vi "MC_7_23a_JW.vi"() -> ()   [LabVIEW 2011]
uses:
  <vilib>/Utility/file.llb/Read From Spreadsheet File (string).vi
  <vilib>/Utility/inputDevices.llb/keyboardAcquire.vi
  <vilib>/Utility/file.llb/Write To Spreadsheet File (DBL).vi
  <vilib>/Utility/file.llb/Write To Spreadsheet File (string).vi
  <vilib>/regexp/Match Regular Expression.xnode
panel:
  out "New: Temp":dbl
  out "XY Graph-Lin":cluster{dbl[], dbl[]}[](graph)
  out "Lin Vd":dbl
  out "Lin-Vg Array-Used":dbl[](array[numeric])
  out "Lin Id-Used":dbl[](array[numeric])
  out "Rec: Temp":dbl
  out "Comments":string
  out "Folder Index":dbl caption="Length"
  out "Current \nRecord":string[](array[string])
  out "Transformer \nHeaders":string[](array[string])
  out "Current Device ID":string
  out "Column":string
  out "Row":string
  out "Rec: Concentration":dbl
  out "Rec: Solvent":string
  out "Rec: Method":string
  in  "?":T1(tab)
  out "Rec: Material":string
  in  "Treatment Concentration (mM):":dbl=30.0
  in  "Surface Treatment:":string
  in  "# Drops*:":dbl=inf
  in  "Solution Temp (C):":dbl=55.0
  in  "Relative Humidity (%):":dbl=nan
  in  "Room Temp (F):":dbl=nan
  in  "Time (s):":dbl=80.0
  out "Accel (RPM/s):":dbl
  in  "RPM:":dbl=1000.0
  in  "Wait Time (s):":dbl=10.0
  in  "Sample #:":dbl=1.0
  in  "Fabricator:":string="Jeremy"
  in  "Data File":path
  out "Data Folder":path
  in  "Image Folder":path
  out "Image File":path=path "D:/UserData/Desktop/Jeremy/WFU/Research/Programs/VI mods/Image Not Found.png"
  in  "Ramp (s):":dbl=3.0
  out "Calc: Off I-Sat":dbl caption="Off I-Sat" format="%#_3e"
  in  "Manuel-Dielectric":bool
  in  "Manuel-Length":bool
  out "Calc: VT-Lin":dbl
  out "New: VT-Lin":dbl
  out "Rec: VT-Lin":dbl caption="VT-Lin" format="%#_3g"
  out "Calc: Trap Density-STS":dbl format="%#_4e"
  out "New: Trap Density-STS":dbl format="%#_4e"
  out "Rec: Trap Density-STS":dbl caption="N-Sat (STS)" format="%#_3e"
  out "Calc: Trap Density-VT":dbl format="%#_4e"
  out "New: Trap Density-VT":dbl format="%#_4e"
  out "Rec: Trap Density-VT":dbl caption="N-Sat (VT)" format="%#_3e"
  out "Calc: Mobility-Lin":dbl format="%#_4e"
  out "New: Mobility-Lin":dbl format="%#_4e"
  out "Rec: Mobility-Lin":dbl caption="Mobility-Lin" format="%#_3e"
  out "Calc: Mobility-Sat":dbl format="%#_4e"
  out "Rec: Length":dbl caption="Length" format="%#_3g"
  out "Rec: Width":dbl caption="Width" format="%#_4g"
  out "Rec: Dielectric (d)":dbl caption="Dielectric (d)" format="%#_3g"
  out "XY Graph":cluster{dbl[], dbl[]}[](graph)
  in  "NumPts":dbl=5.0
  in  "Cancel Button":bool
  in  "Next Button":bool
  in  "Previous Button":bool
  in  "Up Button":bool
  in  "Down Button":bool
  out "Data Name:":string
  in  "Save Changes?":bool
  in  "New: Dielectric":dbl
  in  "New: Length":dbl
  in  "New: Width":dbl
  out "New: Mobility-Sat":dbl format="%#_4e"
  in  "Slide":dbl(slide) step=1.0 scale=-14.3..84.0 scale format="%#_1p"
  in  "Blank Button":bool
  in  "Zoom":i16(slide)=-3 scale=-5.0..5.0
  out "Image Out 2":T2(plugin-control)
  out "Image Out":T2(plugin-control)
  in  "Magnification":u16(ring) items=["5x", "10x", "20x", "50x", "80x"]
  out "Total Width":dbl
  out "Distances":dbl[](array[numeric])
  in  "Undo Button":bool
  in  "Remove Button":bool
  out "Rec: Mobility-Sat":dbl caption="Mobility-Sat" format="%#_3e"
  out "Index":string
  out "Image Name":string
  in  "Export":bool
  out "Calc: VT-Sat":dbl
  out "New: VT-Sat":dbl
  in  "Manual-Width":bool caption="Manual"
  out "XY Graph 2":cluster{dbl[], dbl[]}[](graph)
  in  "Next Button 2":bool
  in  "Previous Button 2":bool
  in  "Slide 2":dbl(slide) step=1.0 scale=-1.0..82.0 scale format="%#_1p"
  out "Calc: STS":dbl
  out "New: STS":dbl
  in  "NumPts 2":dbl=5.0 caption="NumPts"
  out "Rec: VT-Sat":dbl caption="VT-Sat" format="%#_3g"
  out "Rec: STS":dbl caption="STS-Sat" format="%#_3g"
  out "Rec: On/Off":dbl caption="On/Off-Sat" format="%#_3e"
  in  "Save Changes? 2":bool
  in  "Save Changes? 3":bool
  out "Date Recorded":string="Date Recorded" caption="Recorded"
  out "Date Created":string caption="Fabricated"
  out "String":string
  in  "No Image":path=path "D:/UserData/Desktop/Jeremy/WFU/Research/Programs/VI mods/Image Not Found.png"
  in  "Project":path=path "D:/UserData/Desktop/Jeremy/WFU/Research/Programs/Mega Awesome/DeviceData.opj"
  out "Index 2":dbl
  out "Sat Id-Log-Used":dbl[](array[numeric])
  out "Vg Array-Log-Used":dbl[](array[numeric])
  out "ROI Descriptor out":T3 {"Contours"."Type" items=["No Selection", "Point", "Line", "Rectangle", "Oval", "Polygon", "Freehand Region", "Annulus", "Unused2", "Unused3", "Broken Line", "Freehand Line", "Rotated Rectangle"]}
  out "ROI Descriptor":T3 {"Contours"."Type" items=["No Selection", "Point", "Line", "Rectangle", "Oval", "Polygon", "Freehand Region", "Annulus", "Unused2", "Unused3", "Broken Line", "Freehand Line", "Rotated Rectangle"]}
  out "Numeric 3":dbl
  out "Array 6":dbl[][](array[numeric])
  out "Cluster":T4
  out "Array 5":dbl[](array[numeric])
  out "Array 4":dbl[](array[numeric])
  out "Array 3":dbl[](array[numeric])
  out "Numeric 2":dbl
  out "Numeric":dbl
  out "Sat Id-Used":dbl[](array[numeric])
  out "Sat Vg Array-Used":dbl[](array[numeric])
  out "MobVi Index":dbl
  in  "Row Start":dbl=20.0
  # "Data Locations"
  # "Data Location"
  # "Image Location"
  # "Sample Properties"
  # "*     Inf = Full coverage\n   NaN = Unknown or Not Applicable"
  # "Recorded"
  # "Calculated"
  # "Re-Calculated"
  # "Manual"
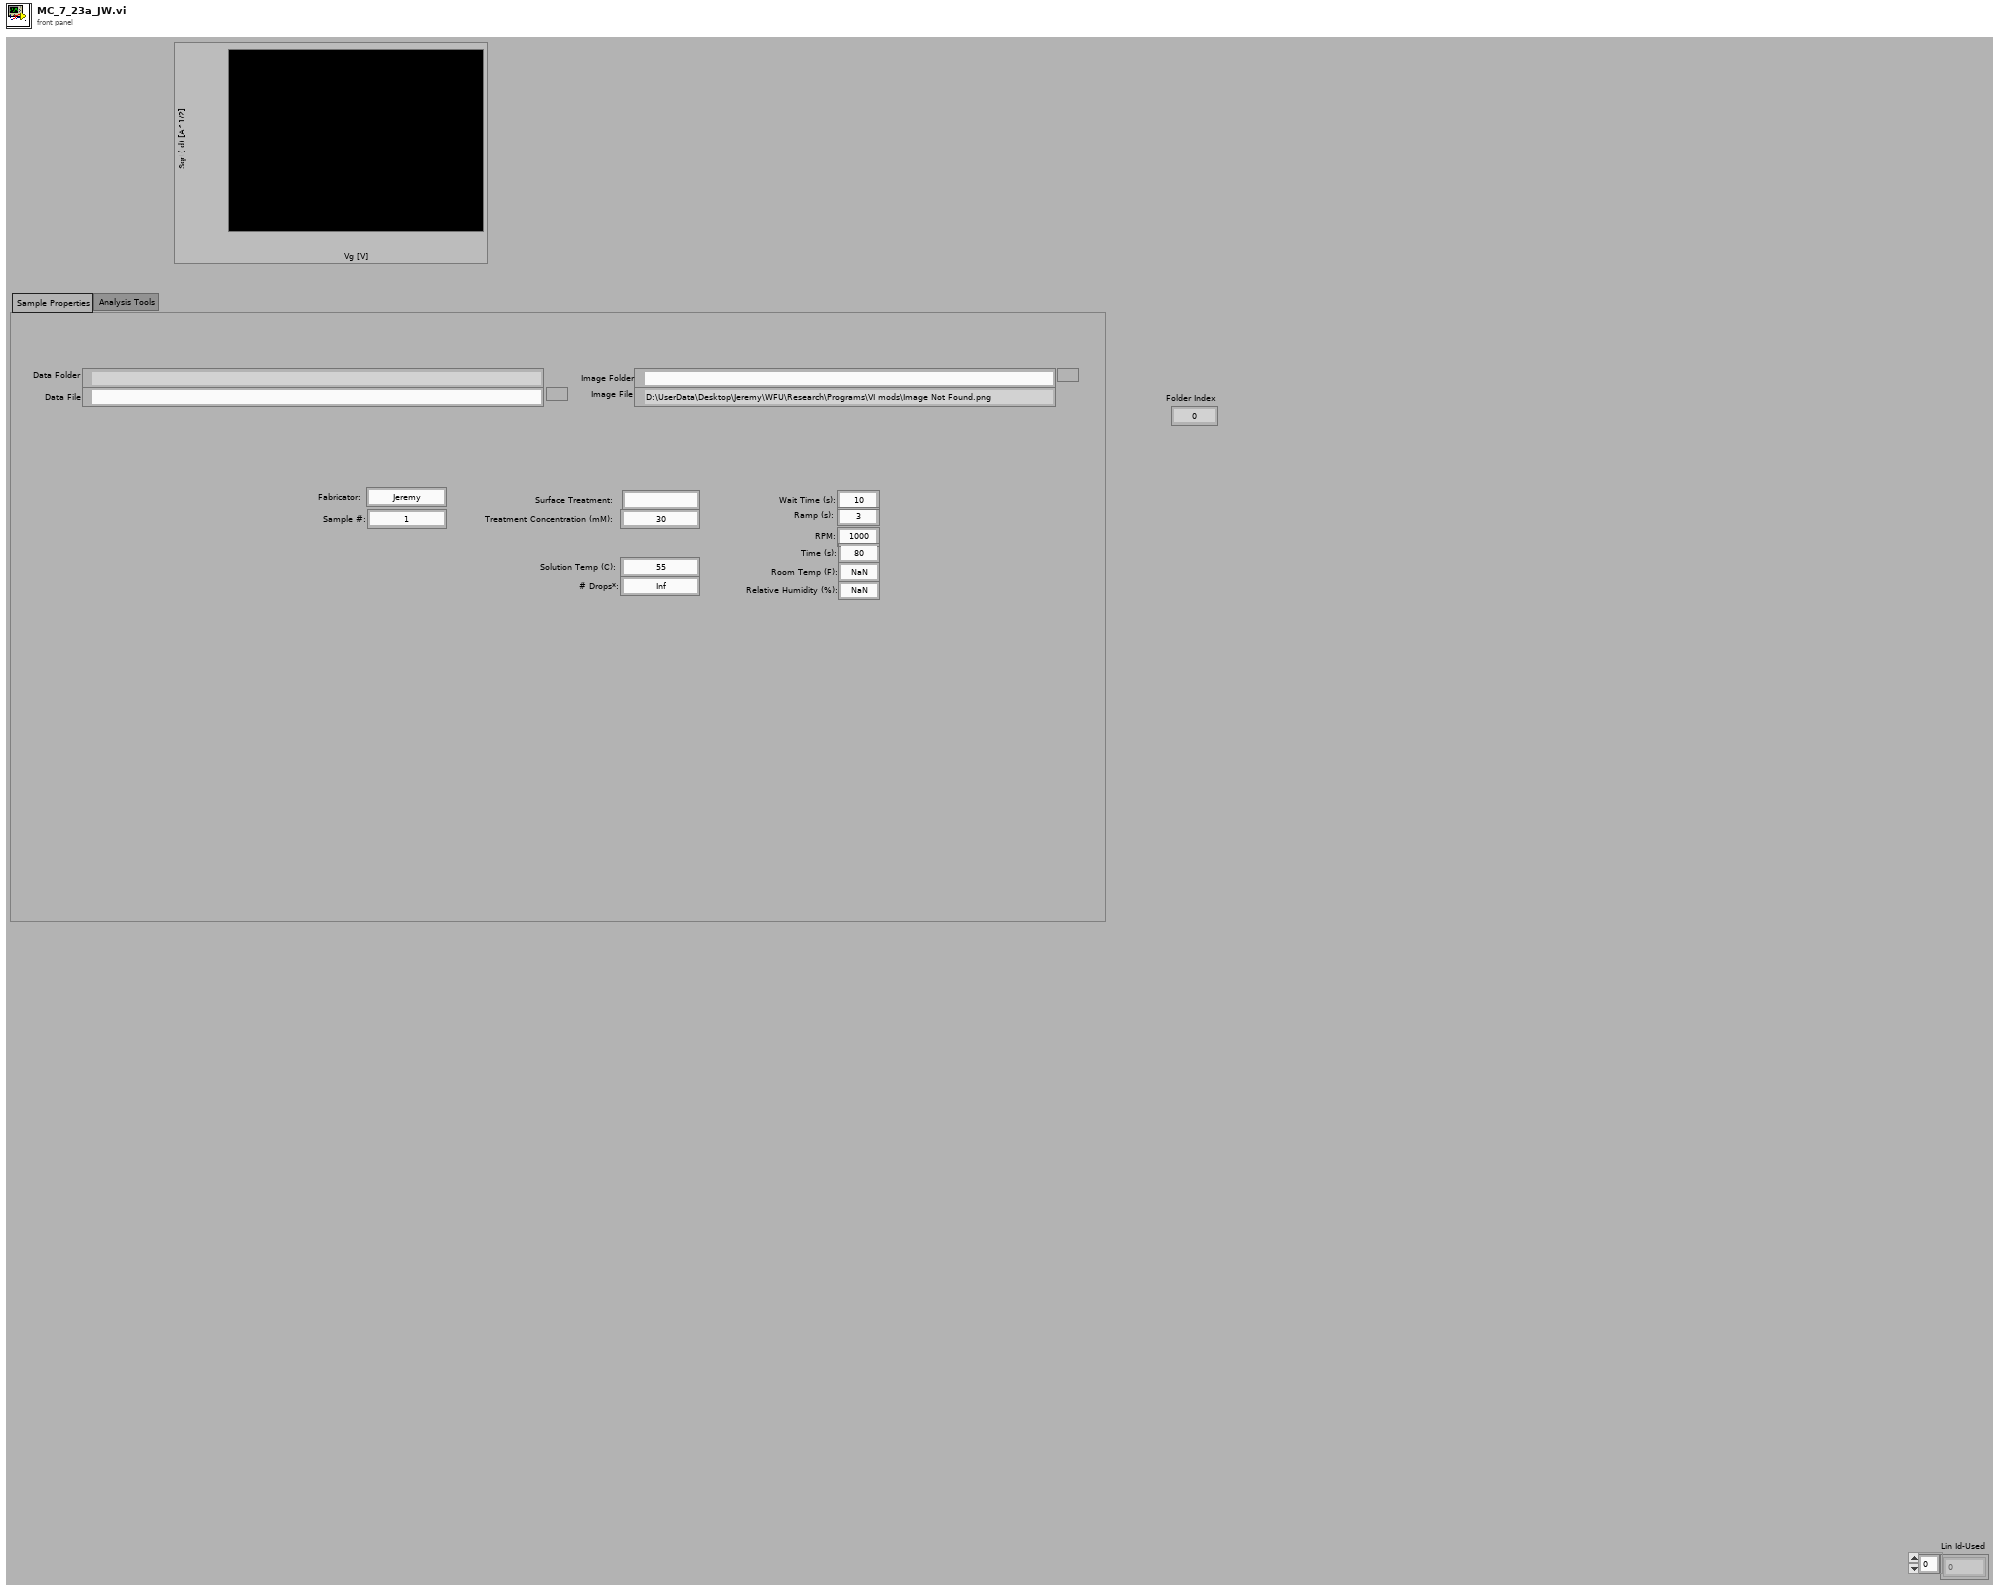
[diagram p1: front panel]
types:
  T1 = enum32{"Sample Properties", "Analysis Tools", "Current Database"}
  T2 = typedef "IMAQ Image.ctl" = refnum<image>
  T3 = typedef "ROI Descriptor" = cluster{"Global Rectangle":i32[], "Contours":cluster{"ID":enum32{"External", "Internal"}, "Type":u32, "Coordinates":i32[]}[]}
  T4 = cluster{"Numeric":dbl, "Numeric 2":dbl, "Numeric 3":dbl, "Numeric 4":dbl}
  T5 = cluster{"Mobility-Sat":dbl, "Moblitity-Lin":dbl, "On/Off":dbl, "Threshold Voltage":dbl, "Onset Voltage":dbl, "STS":dbl, "Trap Density-VT":dbl, "Trap Density-STS":dbl}
  T6 = cluster{"Date Recorded":string, "Index":string, "Length":dbl, "Width":dbl, "Sample Temp":dbl}
  T7 = cluster{"Date Created":string, "Material":string, "Solvent":string, "Concentration":dbl, "Method":string, "Dielectric (nm)":dbl, "Treatment":string, "Comments":string}
  T8 = cluster{"Mobility-Sat":dbl, "Vt-Sat":dbl, "Mobility-Lin":dbl, "Vt-Lin":dbl, "Off I-Sat":dbl, "Off I-Lin":dbl}
  T9 = cluster{"[0]":cluster{dbl[], dbl[]}, "[1]":cluster{dbl[], dbl[]}, "[2]":cluster{dbl[], dbl[]}, "[3]":cluster{dbl[], dbl[]}, "[4]":cluster{dbl[], dbl[]}, "[5]":cluster{dbl[], dbl[]}, "[6]":cluster{dbl[], dbl[]}, "[7]":cluster{dbl[], dbl[]}, "[8]":cluster{dbl[], dbl[]}}
  T10 = cluster{"Global Rectangle":i32[], "Contours":cluster{"Contour Type":u32, "ROI Type":u32, "Points":i32[]}[]}
  T11 = typedef "LVBoundsTypeDef.ctl" = cluster{"Width":u32, "Height":u32}
  T12 = enum16{"0", "1", "2", "3", "4", "5", "6", "7", "8", "9", "A", "B", "C", "D", "E", "F", "G", "H", "I", "J", "K", "L", "M", "N", "O", "P", "Q", "R", "S", "T", "U", "V", "W", "X", "Y", "Z", "F1", "F2", "F3", "F4", "F5", "F6", "F7", "F8", "F9", "F10", "F11", "F12", "F13", "F14", "F15", "ADD", "BACK", "BACKSLASH", "CAPITAL", "COMMA", "DECIMAL", "DELETE", "DIVIDE", "DOWN", "END", "EQUALS", "ESCAPE", "GRAVE (`)", "HOME", "INSERT", "LBRACKET", "LCONTROL", "LEFT", "L ALT", "LSHIFT", "LWIN", "MINUS", "MULTIPLY", "NEXT", "NUMLOCK", "NUMPAD_0", "NUMPAD_1", "NUMPAD_2", "NUMPAD_3", "NUMPAD_4", "NUMPAD_5", "NUMPAD_6", "NUMPAD_7", "NUMPAD_8", "NUMPAD_9", "PAUSE", "PERIOD", "PRIOR (PG UP)", "RBRACKET", "RCONTROL", "RETURN", "RIGHT", "R ALT", "RSHIFT", "RWIN", "SCROLL", "SEMICOLON", "SLASH", "SPACE", "SUBTRACT", "TAB", "UP", "ENTER (num pad)", "' (quote)"}[]
  T13 = enum16{"0", "1", "2", "3", "4", "5", "6", "7", "8", "9", "A", "B", "C", "D", "E", "F", "G", "H", "I", "J", "K", "L", "M", "N", "O", "P", "Q", "R", "S", "T", "U", "V", "W", "X", "Y", "Z", "F1", "F2", "F3", "F4", "F5", "F6", "F7", "F8", "F9", "F10", "F11", "F12", "F13", "F14", "F15", "ADD", "BACK", "BACKSLASH", "CAPITAL", "COMMA", "DECIMAL", "DELETE", "DIVIDE", "DOWN", "END", "EQUALS", "ESCAPE", "GRAVE (`)", "HOME", "INSERT", "LBRACKET", "LCONTROL", "LEFT", "L ALT", "LSHIFT", "LWIN", "MINUS", "MULTIPLY", "NEXT", "NUMLOCK", "NUMPAD_0", "NUMPAD_1", "NUMPAD_2", "NUMPAD_3", "NUMPAD_4", "NUMPAD_5", "NUMPAD_6", "NUMPAD_7", "NUMPAD_8", "NUMPAD_9", "PAUSE", "PERIOD", "PRIOR (PG UP)", "RBRACKET", "RCONTROL", "RETURN", "RIGHT", "R ALT", "RSHIFT", "RWIN", "SCROLL", "SEMICOLON", "SLASH", "SPACE", "SUBTRACT", "TAB", "UP", "ENTER (num pad)", "' (quote)"}
  T14 = cluster{"Contour Type":u32, "ROI Type":u32, "Points":i32[]}[]
  T15 = cluster{i32[], cluster{"Contour Type":u32, "ROI Type":u32, "Points":i32[]}[]}
  T16 = cluster{string, sgl, bool, bool, bool, bool, bool, bool, i32}
  T17 = cluster{i32, cluster{string, sgl, bool, bool, bool, bool, bool, bool, i32}, i32, i32}
  T18 = cluster{"Contour Type":u32, "ROI Type":u32, "Points":i32[]}
  T19 = cluster{"Points[0]":i32, "Points[1]":i32, "Points[2]":i32, "Points[3]":i32, "Points[4]":i32, "Points[5]":i32, "Points[6]":i32, "Points[7]":i32, "Points[8]":i32}
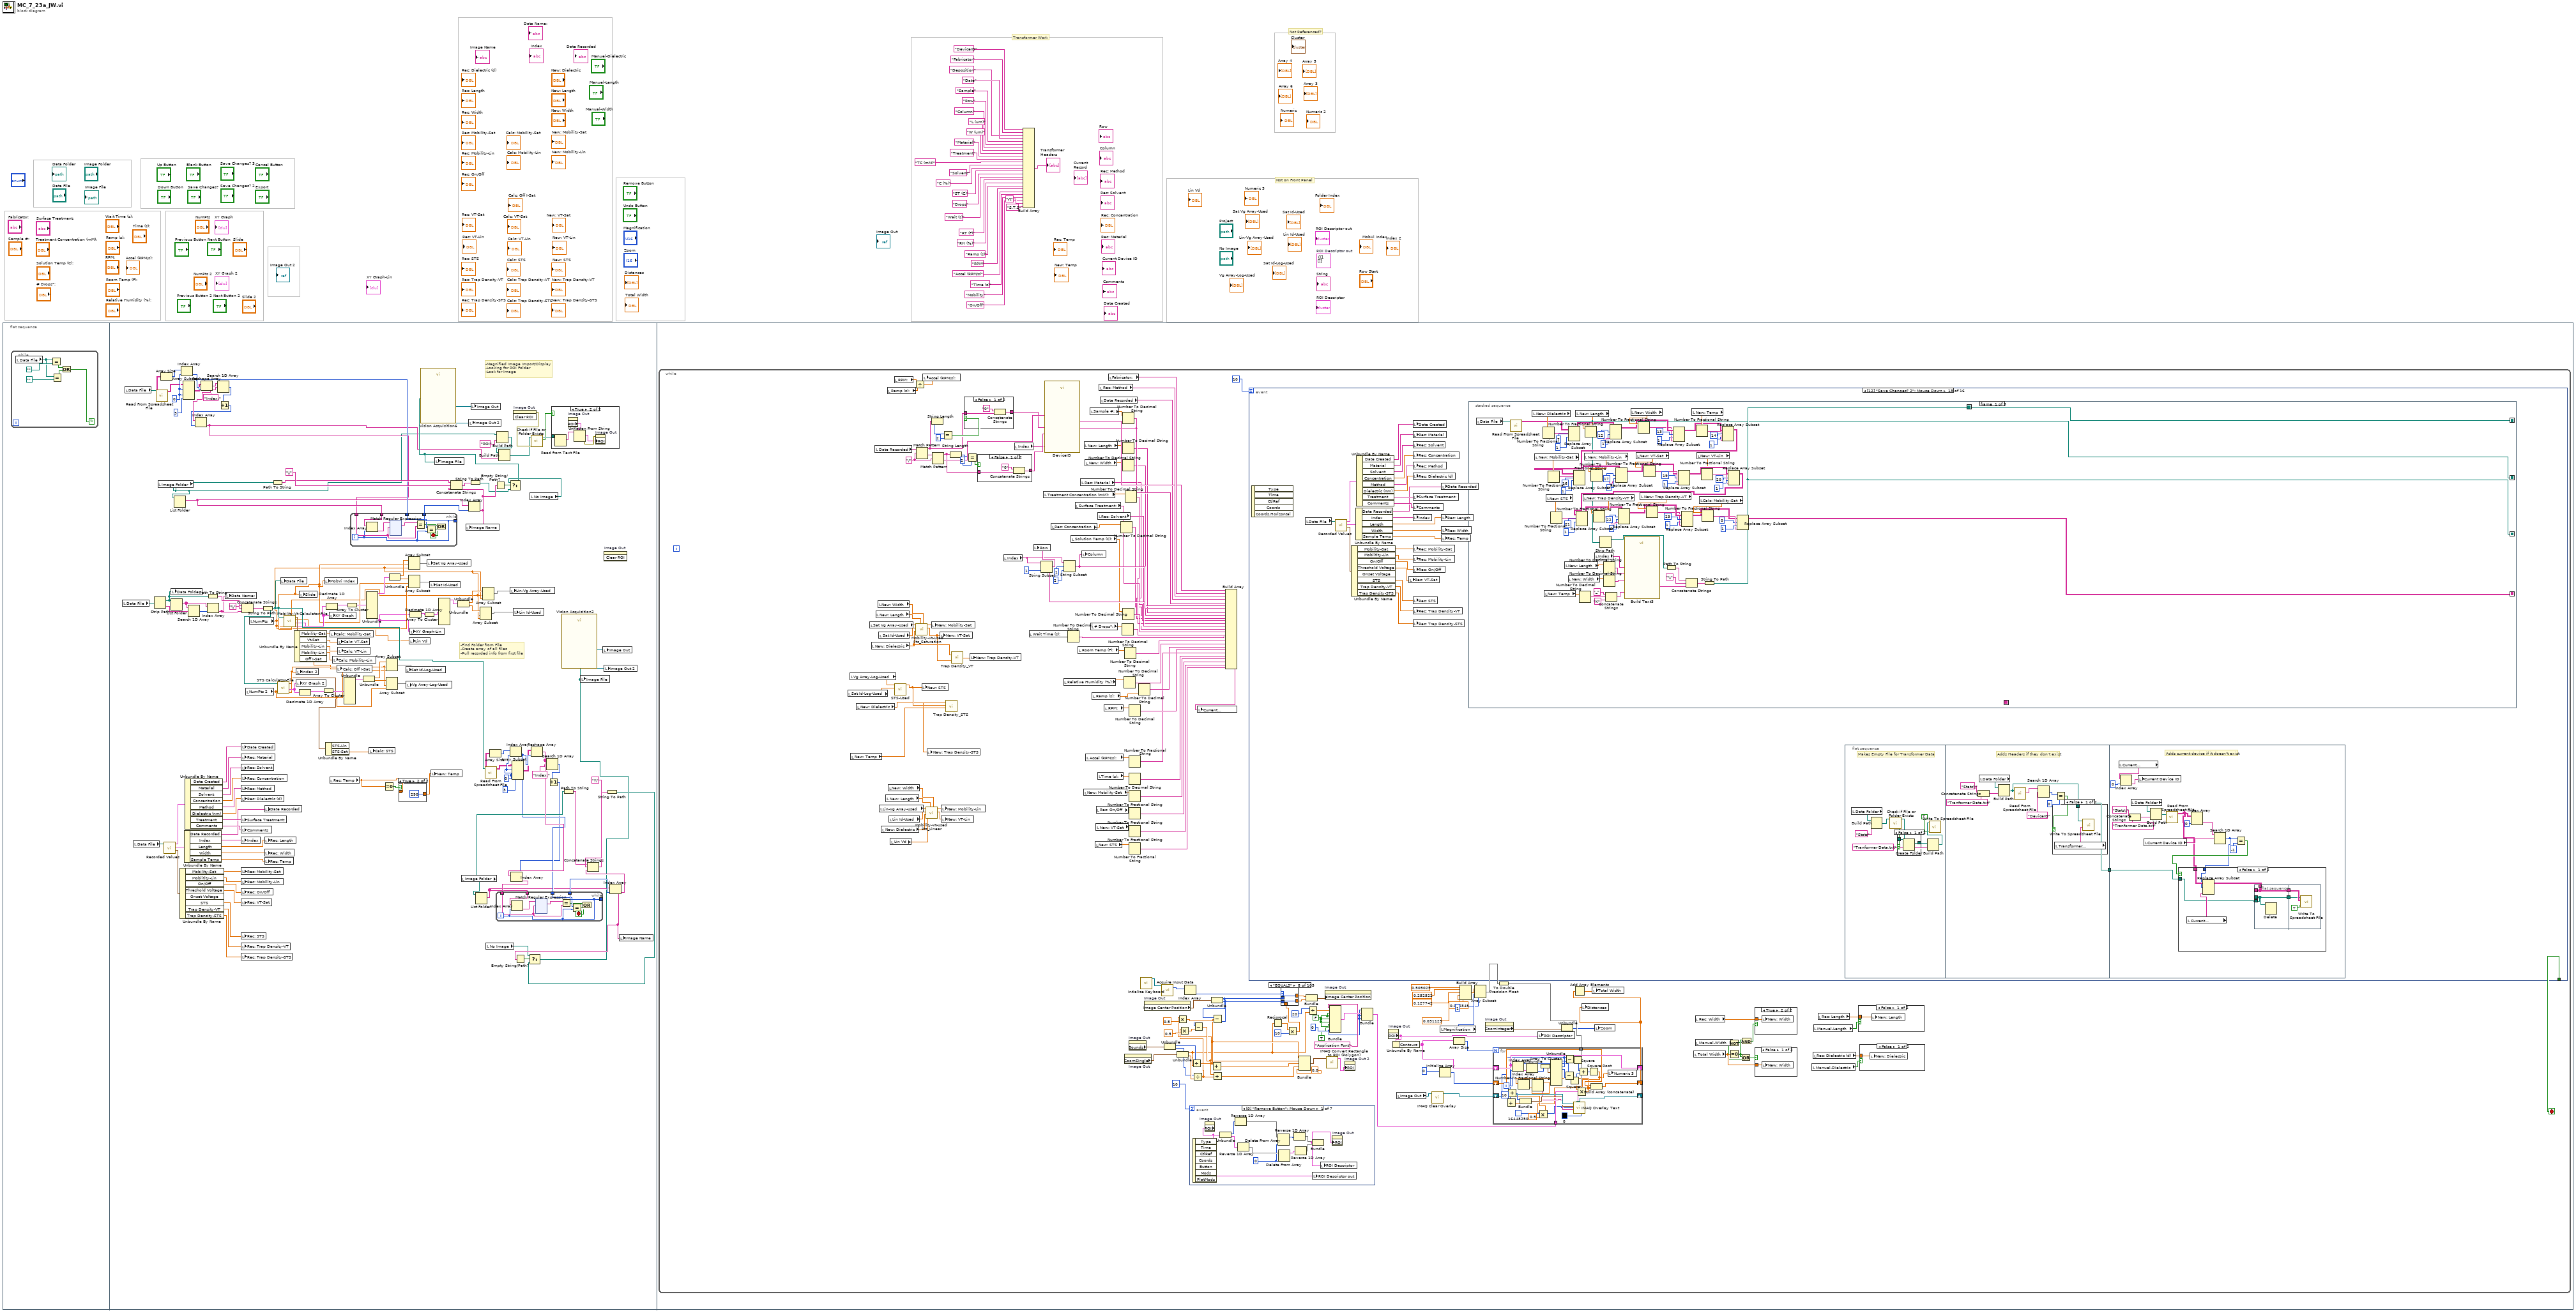
[diagram p0: block diagram]
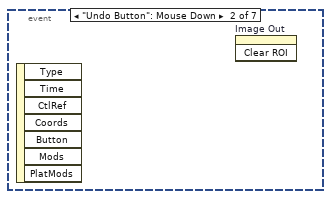
[diagram p10: hidden frame]
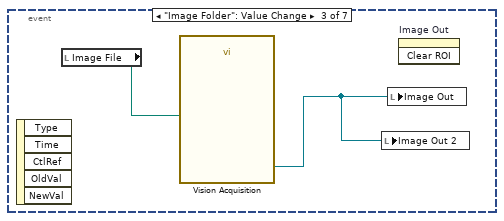
[diagram p11: hidden frame]
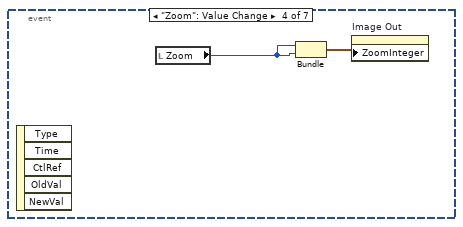
[diagram p12: hidden frame]
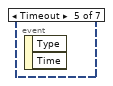
[diagram p13: hidden frame]
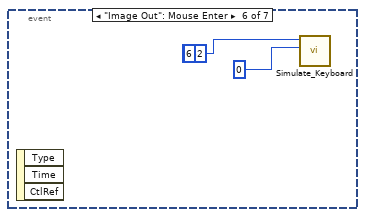
[diagram p14: hidden frame]
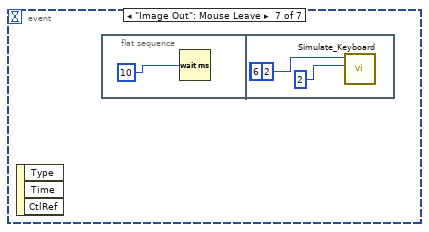
[diagram p15: hidden frame]
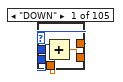
[diagram p16: hidden frame]
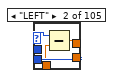
[diagram p17: hidden frame]
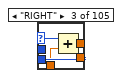
[diagram p18: hidden frame]
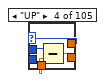
[diagram p19: hidden frame]
diagram:
  (unwired) T3 {"Global Rectangle"=[], "Contours"=[]}  # ROI Descriptor out
  # "Not Referenced?"
  # "Transformer Work"
  # "Not on Front Panel"
  n1 = flat-sequence {
    frame #0 {
      n2 = while {
        stop <- w29 continue-if-true
        n3 = local read "Data File"() -> (w31:path)
        n4 = Equal?(x=w31, y=path "") -> (x = y?=w33:bool)
        n5 = Equal?(x=w31, y=path "") -> (x = y?=w32:bool)
        n6 = Or(x=w33, y=w32) -> (x .or. y?=w29:bool)
      }
    }
    frame #1 {
      w127 = 0
      w151 = 0
      # "-Find Folder from File\n-Create array of all files\n-Pull recorded info from first file"
      # "-Magnified Image Import/Display\n-Looking for ROI Folder\n-Look for Image"
      n7 = local read "Data File"() -> (w131:path)
      n8 = local read "Data File"() -> (w146:path)
      n9 = local read "Data File"() -> (w86:path)
      n10 = Strip Path(path=w131) -> (stripped path=w132:path, name=w118:string)
      n11 = call-poly <vilib>:"Read From Spreadsheet File.vi"("file path (dialog if empty)"=w146) -> ("all rows"=w149:string[][])  [unwired: 6 in, 4 out]
      n12 = local read "Image Folder"() -> (w88:path)
      n13 = Array Size(array=w149) -> (size(s)=w150:i32[])
      n14 = call "Recorded Values.vi"("Path"=w86) -> ("Recorded Char"=w84:T5, "Recorded Prop"=w83:T6, "Fabrication Prop"=w85:T7)  [unwired: 8 in]
      n15 = local write "Data Folder"(w132) -> ()
      n16 = List Folder(path=w132) -> (filenames=w122:string[])  [unwired: 3 in, 3 out]
      n17 = List Folder(path=w88) -> (filenames=w155:string[])  [unwired: 3 in, 3 out]
      n18 = Unbundle By Name(w84) -> ("Mobility-Sat"=w70:dbl, "Moblitity-Lin"=w69:dbl, "On/Off"=w68:dbl, "Threshold Voltage"=w67:dbl, "STS"=w66:dbl, "Trap Density-VT"=w65:dbl, "Trap Density-STS"=w64:dbl)  [unwired: 1 out]
      n19 = Index Array(array=w150, index=w151) -> (element=w157:i32)
      n20 = Array Subset(array=w149, index (row)=w151, index (col)=w151, length (col)=3) -> (w148:string[][])  [unwired: 1 in]
      n21 = Unbundle By Name(w83) -> ("Date Recorded"=w75:string, "Index"=w74:string, "Length"=w73:dbl, "Width"=w72:dbl, "Sample Temp"=w71:dbl)
      n22 = Unbundle By Name(w85) -> ("Date Created"=w63:string, "Material"=w82:string, "Solvent"=w81:string, "Concentration"=w80:dbl, "Method"=w79:string, "Dielectric (nm)"=w78:dbl, "Treatment"=w77:string, "Comments"=w76:string)
      n23 = Search 1D Array(1D array=w122, element=w118) -> (index of element=w121:i32)  [unwired: 1 in]
      n24 = Reshape Array(w148, w157) -> (w162:string[])
      n25 = Path To String(path=w132) -> (string=w117:string)
      n26 = Index Array(array=w122, index=w121) -> (element=w87:string)
      n27 = Search 1D Array(1D array=w162, element="Index:") -> (index of element=w154:i32)  [unwired: 1 in]
      n28 = Increment(x=w154) -> (x+1=w153:i32)
      n29 = Index Array(array=w162, index=w153) -> (element=w89:string)
      n30 = local write "Data Name:"(w87) -> ()
      n31 = local write "Date Created"(w63) -> ()
      n32 = local write "Rec: Material"(w82) -> ()
      n33 = local write "Rec: Solvent"(w81) -> ()
      n34 = local write "Rec: Concentration"(w80) -> ()
      n35 = local write "Rec: Method"(w79) -> ()
      n36 = local write "Rec: Dielectric (d)"(w78) -> ()
      n37 = local write "Surface Treatment:"(w77) -> ()
      n38 = local write "Comments"(w76) -> ()
      n39 = local write "Index"(w74) -> ()
      n40 = local write "Rec: Mobility-Sat"(w70) -> ()
      n41 = local write "Rec: Mobility-Lin"(w69) -> ()
      n42 = local write "Rec: On/Off"(w68) -> ()
      n43 = local write "Rec: VT-Sat"(w67) -> ()
      n44 = local write "Rec: STS"(w66) -> ()
      n45 = local write "Rec: Trap Density-VT"(w65) -> ()
      n46 = local write "Rec: Trap Density-STS"(w64) -> ()
      n47 = Concatenate Strings(w117, "\\", w87) -> (w119:string)
      n48 = local read "NumPts 2"() -> (w54:dbl)
      n49 = local read "NumPts"() -> (w44:dbl)
      n50 = String To Path(string=w119) -> (path=w62:path)
      n51 = local write "Date Recorded"(w75) -> ()
      n52 = local write "Rec: Length"(w73) -> ()
      n53 = local write "Rec: Width"(w72) -> ()
      n54 = local write "Rec: Temp"(w71) -> ()
      n55 = Path To String(path=w88) -> (string=w159:string)
      n56 = call "STS Calculator-File.vi"("NumPts"=w54, "Path"=w62) -> ("STS Index-Sat"=w52:dbl, "XY Graph-Sat"=w53:cluster{dbl[], dbl[]}[], "Ouput"=w51:cluster{"STS-Sat":dbl, "STS-Lin":dbl})  [unwired: 5 in, 2 out]
      n57 = local write "Data File"(w62) -> ()
      n58 = call "Mobility-Vt Calculator-File.vi"("NumPts"=w44, "Path"=w62) -> ("XY Graph-Sat"=w56:cluster{dbl[], dbl[]}[], "XY Graph-Lin"=w39:cluster{dbl[], dbl[]}[], "Lin Vd"=w40:dbl, "Output"=w57:T8, "Index-Sat"=w55:dbl, "Index-Lin"=w43:dbl)  [unwired: 4 in]
      n59 = Unbundle By Name(w57) -> ("Mobility-Sat"=w61:dbl, "Vt-Sat"=w60:dbl, "Mobility-Lin"=w59:dbl, "Mobility-Lin"=w58:dbl, "Off I-Sat"=w35:dbl)
      n60 = local write "Index 2"(w52) -> ()
      n61 = local write "XY Graph 2"(w53) -> ()
      n62 = local write "Slide"(w55) -> ()
      n63 = Decimate 1D Array(w53) -> (w109:cluster{dbl[], dbl[]}[])  [unwired: 1 out]
      n64 = Array To Cluster(array=w109) -> (cluster=w111:T9)
      n65 = local write "MobVi Index"(w55) -> ()
      n66 = Unbundle By Name(w51) -> ("STS-Sat"=w50:dbl)  [unwired: 1 out]
      n67 = Decimate 1D Array(w56) -> (w145:cluster{dbl[], dbl[]}[])  [unwired: 1 out]
      n68 = local write "XY Graph"(w56) -> ()
      n69 = local read "Rec: Temp"() -> (w37:dbl)
      n70 = local write "Calc: Mobility-Sat"(w61) -> ()
      n71 = local write "Calc: Mobility-Lin"(w58) -> ()
      n72 = local write "Calc: Off I-Sat"(w35) -> ()
      n73 = local write "Calc: VT-Sat"(w60) -> ()
      n74 = local write "Calc: VT-Lin"(w59) -> ()
      n75 = Unbundle(w111) -> ("[0]"=w110:cluster{dbl[], dbl[]})  [unwired: 8 out]
      n76 = Array To Cluster(array=w145) -> (cluster=w143:T9)
      n77 = while {
        tunnel: w155 -> [w297]
        tunnel: w89 -> [w295]
        tunnel: [w294] -> _
        tunnel: [w294] -> w156
        tunnel: w157 -> [w293]
        i -> [w294]
        stop <- w290 stop-if-true
        n78 = Index Array(array=w297, index=w294) -> (element=w298:string)
        n79 = xnode "Match Regular Expression"("input string"=w298, "regular expression"=w295) -> ("whole match"=w296:string)  [unwired: 4 in, 4 out]
        n80 = Equal?(x=w296, y=w295) -> (x = y?=w292:bool)
        n81 = Equal?(x=w293, y=w294) -> (x = y?=w291:bool)
        n82 = Or(x=w292, y=w291) -> (x .or. y?=w290:bool)
      }
      n83 = Unbundle(w110) -> (w107:dbl[], w106:dbl[])
      n84 = Unbundle(w143) -> ("[0]"=w144:cluster{dbl[], dbl[]})  [unwired: 8 out]
      n85 = local write "Calc: STS"(w50) -> ()
      n86 = Equal To 0?(x=w37) -> (x = 0?=w38:bool)
      n87 = Array Subset(array=w107, index=w52, length=w54) -> (w114:dbl[])
      n88 = Array Subset(array=w106, index=w52, length=w54) -> (w113:dbl[])
      n89 = Unbundle(w144) -> (w108:dbl[], w112:dbl[])
      n90 = case shown="True" w38 {
        tunnel: [w163 290] -> w36
        tunnel: w37 -> [w163 _]
        frame False {
        }
        frame True {
        }
      }
      n91 = local write "Sat Id-Log-Used"(w114) -> ()
      n92 = local write "Vg Array-Log-Used"(w113) -> ()
      n93 = Array Subset(array=w108, index=w55, length=w44) -> (w115:dbl[])
      n94 = Array Subset(array=w112, index=w55, length=w44) -> (w116:dbl[])
      n95 = local write "Lin Vd"(w40) -> ()
      n96 = Decimate 1D Array(w39) -> (w49:cluster{dbl[], dbl[]}[])  [unwired: 1 out]
      n97 = local write "XY Graph-Lin"(w39) -> ()
      n98 = Array To Cluster(array=w49) -> (cluster=w48:T9)
      n99 = local write "Sat Vg Array-Used"(w115) -> ()
      n100 = local write "Sat Id-Used"(w116) -> ()
      n101 = local write "New: Temp"(w36) -> ()
      n102 = Unbundle(w48) -> ("[0]"=w47:cluster{dbl[], dbl[]})  [unwired: 8 out]
      n103 = Unbundle(w47) -> (w46:dbl[], w45:dbl[])
      n104 = local read "Image Folder"() -> (w138:path)
      n105 = Index Array(array=w155, index=w156) -> (element=w105:string)
      n106 = Concatenate Strings(w159, "\\", w105) -> (w160:string)
      n107 = local write "Image Name"(w105) -> ()
      n108 = String To Path(string=w160) -> (path=w103:path)
      n109 = List Folder(path=w138) -> (filenames=w134:string[])  [unwired: 3 in, 3 out]
      n110 = Array Subset(array=w45, index=w43, length=w44) -> (w41:dbl[])
      n111 = Array Subset(array=w46, index=w43, length=w44) -> (w42:dbl[])
      n112 = call-poly <vilib>:"Read From Spreadsheet File.vi"("file path (dialog if empty)"=w62) -> ("all rows"=w125:string[][])  [unwired: 6 in, 4 out]
      n113 = local read "No Image"() -> (w97:path)
      n114 = Array Size(array=w125) -> (size(s)=w126:i32[])
      n115 = Empty String/Path?(string/path=w105) -> (empty?=w104:bool)
      n116 = Build Path(base path=w88, name or relative path="ROI") -> (appended path=w91:path)
      n117 = Build Path(base path=w91, name or relative path=w89) -> (appended path=w90:path)
      n118 = Index Array(array=w126, index=w127) -> (element=w137:i32)
      n119 = local write "Lin-Vg Array-Used"(w42) -> ()
      n120 = Array Subset(array=w125, index (row)=w127, index (col)=w127, length (col)=3) -> (w124:string[][])  [unwired: 1 in]
      n121 = local write "Lin Id-Used"(w41) -> ()
      n122 = invoke on="Image Out" class="ImageControl" method="Clear ROI"() -> (error out=w95:errorcluster)  [unwired: 3 in, 2 out]
      n123 = local read "No Image"() -> (w96:path)
      n124 = Select(t=w96, s=w104, f=w103) -> (s? t:f=w102:path)
      n125 = call "Vision Acquisition6"("Image Path"=w102) -> ("Image Out"=w158:T2)  [unwired: 25 in, 1 out]
      n126 = local write "Image File"(w102) -> ()
      n127 = local write "Image Out 2"(w158) -> ()
      n128 = local write "Image Out"(w158) -> ()
      n129 = call <vilib>:"Check if File or Folder Exists.vi"("error in (no error)"=w95, "path"=w90) -> ("file or folder exists?"=w93:bool, "dup path"=w94:path)  [unwired: 7 in, 1 out]
      n130 = Reshape Array(w124, w137) -> (w142:string[])
      n131 = Search 1D Array(1D array=w142, element="Index:") -> (index of element=w130:i32)  [unwired: 1 in]
      n132 = Increment(x=w130) -> (x+1=w129:i32)
      n133 = Index Array(array=w142, index=w129) -> (element=w135:string)
      n134 = while {
        tunnel: w134 -> [w177]
        tunnel: w135 -> [w175]
        tunnel: [w174] -> _
        tunnel: [w174] -> w136
        tunnel: w137 -> [w173]
        i -> [w174]
        stop <- w170 stop-if-true
        n135 = Index Array(array=w177, index=w174) -> (element=w178:string)
        n136 = xnode "Match Regular Expression"("input string"=w178, "regular expression"=w175) -> ("whole match"=w176:string)  [unwired: 4 in, 4 out]
        n137 = Equal?(x=w176, y=w175) -> (x = y?=w172:bool)
        n138 = Equal?(x=w173, y=w174) -> (x = y?=w171:bool)
        n139 = Or(x=w172, y=w171) -> (x .or. y?=w170:bool)
      }
      n140 = case shown="True" w93 {
        tunnel: w94 -> [_ w165]
        frame False {
        }
        frame True {
          n141 = Read from Text File(file (use dialog)=w165) -> (text=w169:string)  [unwired: 3 in, 3 out]
          n142 = property on="Image Out" class="ImageControl"() -> ("ROI"=w166:T10)  [unwired: 2 in, 2 out]
          n143 = Unflatten From String(type=w166, binary string=w169) -> (value=w167:T10, error out=w168:errorcluster)  [unwired: 3 in, 1 out]
          n144 = property on="Image Out" class="ImageControl"(error in=w168, "ROI"=w167) -> ()  [unwired: 1 in, 2 out]
        }
      }
      n145 = Path To String(path=w138) -> (string=w139:string)
      n146 = invoke on="Image Out" class="ImageControl" method="Clear ROI"() -> ()  [unwired: 3 in, 3 out]
      n147 = Index Array(array=w134, index=w136) -> (element=w100:string)
      n148 = Empty String/Path?(string/path=w100) -> (empty?=w101:bool)
      n149 = Concatenate Strings(w139, "\\", w100) -> (w140:string)
      n150 = String To Path(string=w140) -> (path=w99:path)
      n151 = Select(t=w97, s=w101, f=w99) -> (s? t:f=w98:path)
      n152 = call "Vision Acquisition2"("Image Path"=w98) -> ("Image Out"=w133:T2)  [unwired: 25 in, 1 out]
      n153 = local write "Image File"(w98) -> ()
      n154 = local write "Image Out"(w133) -> ()
      n155 = local write "Image Out 2"(w133) -> ()
      n156 = local write "Image Name"(w100) -> ()
    }
    frame #2 {
      n157 = while {
        stop <- w573 stop-if-true
        w469 = "/"
        w523 = FALSE
        w521 = 0
        n158 = local read "Sat Id-Log-Used"() -> (w426:dbl[])
        n159 = local read "Vg Array-Log-Used"() -> (w425:dbl[])
        n160 = local read "New: Temp"() -> (w410:dbl)
        n161 = local read "New: Dielectric"() -> (w415:dbl)
        n162 = local read "Sat Vg Array-Used"() -> (w428:dbl[])
        n163 = local read "New: Dielectric"() -> (w412:dbl)
        n164 = local read "Date Recorded"() -> (w472:string)
        n165 = local read "New: Length"() -> (w429:dbl)
        n166 = local read "New: Width"() -> (w431:dbl)
        n167 = local read "Sat Id-Used"() -> (w427:dbl[])
        n168 = local read "Lin-Vg Array-Used"() -> (w422:dbl[])
        n169 = local read "New: Dielectric"() -> (w419:dbl)
        n170 = local read "New: Length"() -> (w421:dbl)
        n171 = local read "Ramp (s):"() -> (w439:dbl)
        n172 = local read "New: Width"() -> (w418:dbl)
        n173 = local read "Lin Id-Used"() -> (w423:dbl[])
        n174 = local read "Lin Vd"() -> (w417:dbl)
        n175 = local read "RPM:"() -> (w440:dbl)
        n176 = call "STS-Used.vi"("Id Used"=w426, "Vg-Used"=w425) -> ("STS"=w416:dbl)  [unwired: 9 in]
        n177 = Divide(x=w440, y=w439) -> (x/y=w438:dbl)
        n178 = call "Mobility-Vt-Used Pts_Saturation.vi"("Width"=w431, "Length"=w429, "Dielectric (d)"=w412, "Sat Id Used"=w427, "Vg Used"=w428) -> ("Vt"=w413:dbl, "Mobility"=w430:dbl)  [unwired: 4 in, 1 out]
        n179 = Match Pattern(string=w472, regular expression=w469) -> (before substring=w463:string, after substring=w470:string)  [unwired: 1 in, 2 out]
        n180 = local write "New: STS"(w416) -> ()
        n181 = local write "Accel (RPM/s):"(w438) -> ()
        n182 = call "Mobility-Vt-Used Pts_Linear.vi"("Width"=w418, "Length"=w421, "Vd"=w417, "Dielectric (d)"=w419, "Sat Id Used"=w423, "Vg Used"=w422) -> ("Vt"=w424:dbl, "Mobility"=w420:dbl)  [unwired: 3 in, 1 out]
        n183 = String Length(string=w463) -> (length=w466:i32)
        n184 = local write "New: Mobility-Sat"(w430) -> ()
        n185 = Match Pattern(string=w470, regular expression=w469) -> (before substring=w457:string, after substring=w468:string)  [unwired: 1 in, 2 out]
        n186 = local write "New: VT-Sat"(w413) -> ()
        n187 = local write "New: Mobility-Lin"(w420) -> ()
        n188 = local write "New: VT-Lin"(w424) -> ()
        n189 = Equal?(x=w466, y=2) -> (x = y?=w464:bool)
        n190 = call "Trap Density_STS.vi"("Temp (T) [K]"=w410, "S.T.S. (S)"=w416, "Dielectric"=w415) -> ("Trap Density (N)"=w414:dbl)  [unwired: 8 in]
        n191 = local write "New: Trap Density-STS"(w414) -> ()
        n192 = String Length(string=w457) -> (length=w459:i32)
        n193 = call "Trap Density_VT.vi"("VT"=w413, "Dielectric"=w412) -> ("Trap Density-VT"=w411:dbl)
        n194 = case shown="False" w464 {
          tunnel: w463 -> [w581 w583]
          tunnel: [w580 w583] -> w462
          frame False {
            n195 = Concatenate Strings("0", w581) -> (w580:string)
          }
          frame True {
          }
        }
        n196 = Equal?(x=w459, y=2) -> (x = y?=w461:bool)
        n197 = local write "New: Trap Density-VT"(w411) -> ()
        n198 = case shown="False" w461 {
          tunnel: w457 -> [w577 w579]
          tunnel: [w576 w579] -> w458
          frame False {
            n199 = Concatenate Strings("0", w577) -> (w576:string)
          }
          frame True {
          }
        }
        n200 = local read "Index"() -> (w442:string)
        n201 = local read "Index"() -> (w456:string)
        n202 = local read "Wait Time (s):"() -> (w502:dbl)
        n203 = String Subset(string=w442, length (rest)=1) -> (substring=w497:string)  [unwired: 1 in]
        n204 = local write "Row"(w497) -> ()
        n205 = local read "Treatment Concentration (mM):"() -> (w450:dbl)
        n206 = local read "Rec: Concentration"() -> (w437:dbl)
        n207 = local read "Relative Humidity (%):"() -> (w447:dbl)
        n208 = String Subset(string=w442, offset (0)=1, length (rest)=2) -> (substring=w498:string)
        n209 = Number To Decimal String(number=w502) -> (decimal integer string=w503:string)  [unwired: 1 in]
        n210 = local read "Solution Temp (C):"() -> (w491:dbl)
        n211 = local read "Surface Treatment:"() -> (w449:string)
        n212 = local read "Room Temp (F):"() -> (w495:dbl)
        n213 = local read "Rec: Material"() -> (w445:string)
        n214 = local write "Column"(w498) -> ()
        n215 = local read "New: Mobility-Sat"() -> (w484:dbl)
        n216 = local read "New: Length"() -> (w455:dbl)
        n217 = local read "New: Width"() -> (w454:dbl)
        n218 = local read "Accel (RPM/s):"() -> (w482:dbl)
        n219 = local read "Sample #:"() -> (w474:dbl)
        n220 = local read "# Drops*:"() -> (w492:dbl)
        n221 = local read "Ramp (s):"() -> (w500:dbl)
        n222 = local read "New: STS"() -> (w476:dbl)
        n223 = local read "New: VT-Sat"() -> (w478:dbl)
        n224 = local read "Rec: On/Off"() -> (w480:dbl)
        n225 = local read "Rec: Solvent"() -> (w451:string)
        n226 = local read "Time (s):"() -> (w487:dbl)
        n227 = local read "Rec: Method"() -> (w475:string)
        n228 = local read "Date Recorded"() -> (w471:string)
        n229 = local read "RPM:"() -> (w488:dbl)
        n230 = local read "Fabricator:"() -> (w496:string)
        n231 = Number To Decimal String(number=w437) -> (decimal integer string=w436:string)  [unwired: 1 in]
        n232 = Number To Decimal String(number=w492) -> (decimal integer string=w493:string)  [unwired: 1 in]
        n233 = Number To Decimal String(number=w474) -> (decimal integer string=w467:string)  [unwired: 1 in]
        n234 = call "DeviceID"("Sample"=w467, "Year"=w468, "Month"=w462, "Day"=w458, "Index"=w456) -> ("Result"=w473:string)  [unwired: 9 in, 1 out]
        n235 = Number To Decimal String(number=w455) -> (decimal integer string=w453:string)  [unwired: 1 in]
        n236 = Number To Decimal String(number=w454) -> (decimal integer string=w452:string)  [unwired: 1 in]
        n237 = Number To Decimal String(number=w491) -> (decimal integer string=w490:string)  [unwired: 1 in]
        n238 = Number To Decimal String(number=w447) -> (decimal integer string=w446:string)  [unwired: 1 in]
        n239 = Number To Decimal String(number=w495) -> (decimal integer string=w494:string)  [unwired: 1 in]
        n240 = property on="Image Out" class="ImageControl"() -> ("ZoomSingle"=w541:cluster{"X":sgl, "Y":sgl})  [unwired: 2 in, 2 out]
        n241 = Number To Decimal String(number=w450) -> (decimal integer string=w448:string)  [unwired: 1 in]
        n242 = property on="Image Out" class="ImageControl"() -> ("Bounds"=w542:T11)  [unwired: 2 in, 2 out]
        n243 = Number To Decimal String(number=w488) -> (decimal integer string=w489:string)  [unwired: 1 in]
        n244 = Number To Fractional String(number=w482) -> (F-format string=w483:string)  [unwired: 3 in]
        n245 = Number To Decimal String(number=w487) -> (decimal integer string=w486:string)  [unwired: 1 in]
        n246 = Number To Fractional String(number=w484) -> (F-format string=w485:string)  [unwired: 3 in]
        n247 = Number To Fractional String(number=w480) -> (F-format string=w481:string)  [unwired: 3 in]
        n248 = Number To Fractional String(number=w478) -> (F-format string=w479:string)  [unwired: 3 in]
        n249 = Number To Fractional String(number=w476) -> (F-format string=w477:string)  [unwired: 3 in]
        n250 = Number To Decimal String(number=w500) -> (decimal integer string=w501:string)  [unwired: 1 in]
        n251 = call <vilib>:"Intialize Keyboard.vi"() -> ("device ID"=w553:refnum<k1>)  [unwired: 10 in, 1 out]
        n252 = property on="Image Out" class="ImageControl"() -> ("Image Center Position"=w548:cluster{"X":u32, "Y":u32})  [unwired: 2 in, 2 out]
        n253 = call-poly <vilib>:"Acquire Input Data.vi"("device ID"=w553) -> ("keys pressed"=w552:T12)  [unwired: 16 in, 2 out]
        n254 = Unbundle(w542) -> ("Width"=w539:u32, "Height"=w538:u32)
        n255 = Unbundle(w541) -> ("X"=w516:sgl, "Y"=w540:sgl)
        n256 = Index Array(array=w552) -> (element=w556:T13)  [unwired: 1 in]
        n257 = event shown="[0] \"Remove Button\": Mouse Down" {
          selector: _ -> [_ _ _ _ _ _ _]
          dyn-events: _ -> [_ _ _ _ _ _ _]
          timeout: 10 -> [_ _ _ _ _ _ _]
          event "Remove Button": Mouse Down {
            w588 = 0
            n258 = event-data() -> ()  [unwired: 1 in, 7 out]
            n259 = property on="Image Out" class="ImageControl"() -> ("ROI"=w586:T10)  [unwired: 2 in, 2 out]
            n260 = Unbundle(w586) -> ("Global Rectangle"=w589:i32[], "Contours"=w591:T14)
            n261 = Reverse 1D Array(array=w589) -> (reversed array=w590:i32[])
            n262 = Reverse 1D Array(array=w591) -> (reversed array=w592:T14)
            n263 = Delete From Array(array=w590, index=w588) -> (array with subset deleted=w593:i32[])  [unwired: 1 in, 1 out]
            n264 = Delete From Array(array=w592, index=w588) -> (array with subset deleted=w594:T14)  [unwired: 1 in, 1 out]
            n265 = Reverse 1D Array(array=w593) -> (reversed array=w595:i32[])
            n266 = Reverse 1D Array(array=w594) -> (reversed array=w596:T14)
            n267 = Bundle(w595, w596) -> (w587:T15)  [unwired: 1 in]
            n268 = local write "ROI Descriptor out"(w586) -> ()
            n269 = local write "ROI Descriptor"(w587) -> ()
            n270 = property on="Image Out" class="ImageControl"("ROI"=w587) -> ()  [unwired: 2 in, 2 out]
          }
          event "Undo Button": Mouse Down {
            n271 = event-data() -> ()  [unwired: 1 in, 7 out]
            n272 = invoke on="Image Out" class="ImageControl" method="Clear ROI"() -> ()  [unwired: 3 in, 3 out]
          }
          event "Image Folder": Value Change {
            n273 = event-data() -> ()  [unwired: 1 in, 5 out]
            n274 = local read "Image File"() -> (w598:path)
            n275 = call "Vision Acquisition"("Image Path"=w598) -> ("Image Out"=w597:T2)  [unwired: 25 in, 1 out]
            n276 = local write "Image Out 2"(w597) -> ()
            n277 = local write "Image Out"(w597) -> ()
            n278 = invoke on="Image Out" class="ImageControl" method="Clear ROI"() -> ()  [unwired: 3 in, 3 out]
          }
          event "Zoom": Value Change {
            n279 = event-data() -> ()  [unwired: 1 in, 5 out]
            n280 = local read "Zoom"() -> (w599:i16)
            n281 = Bundle("Zoom"=w599, "Zoom"=w599) -> (w600:cluster{"Zoom":i16, "Zoom":i16})  [unwired: 1 in]
            n282 = property on="Image Out" class="ImageControl"("ZoomInteger"=w600) -> ()  [unwired: 2 in, 2 out]
          }
          event Timeout {
            n283 = event-data() -> ()  [unwired: 1 in, 2 out]
          }
          event "Image Out": Mouse Enter {
            (unwired) 6
            n284 = event-data() -> ()  [unwired: 1 in, 3 out]
            n285 = call "Simulate_Keyboard.vi"("Action"=0, "Virtual Key"=162) -> ()  [unwired: 7 in, 1 out]
          }
          event "Image Out": Mouse Leave {
            n286 = event-data() -> ()  [unwired: 1 in, 3 out]
            n287 = flat-sequence {
              frame #0 {
                n288 = Wait (ms)(milliseconds to wait=10) -> ()  [unwired: 1 out]
              }
              frame #1 {
                (unwired) 6
                n289 = call "Simulate_Keyboard.vi"("Action"=2, "Virtual Key"=162) -> ()  [unwired: 7 in, 1 out]
              }
            }
          }
        }
        n290 = Divide(x=w539, y=w516) -> (x/y=w529:sgl)
        n291 = Multiply(x=w529, y=0.5) -> (x*y=w535:dbl)
        n292 = Divide(x=w538, y=w540) -> (x/y=w528:sgl)
        n293 = Multiply(x=w528, y=0.5) -> (x*y=w534:dbl)
        n294 = Unbundle(w548) -> ("X"=w530:u32, "Y"=w531:u32)
        n295 = Subtract(x=w531, y=w534) -> (x-y=w532:dbl)
        n296 = Subtract(x=w530, y=w535) -> (x-y=w533:dbl)
        n297 = Add(x=w533, y=w529) -> (x+y=w547:dbl)
        n298 = Add(x=w532, y=w528) -> (x+y=w546:dbl)
        n299 = Build Array(w473, w496, w475, w471, w467, w497, w498, w453, w452, w445, w449, w448, w451, w436, w490, w493, w503, w494, w446, w501, w489, w483, w486, w485, w481, w479, w477) -> (w499:string[])
        n300 = local write "Current \nRecord"(w499) -> ()
        n301 = event shown="[12] \"Save Changes? 2\": Mouse Down" {
          selector: _ -> [_ _ _ _ _ _ _ _ _ _ _ _ _ _ _ _]
          dyn-events: _ -> [_ _ _ _ _ _ _ _ _ _ _ _ _ _ _ _]
          timeout: 10 -> [_ _ _ _ _ _ _ _ _ _ _ _ _ _ _ _]
          tunnel: [_ _ _ _ _ _ _ _ _ _ _ _ _ TRUE _ TRUE] -> w573
          event Timeout {
            n302 = event-data() -> ()  [unwired: 1 in, 2 out]
          }
          event "Down Button": Mouse Down {
            w936 = 0
            n303 = event-data() -> ()  [unwired: 1 in, 7 out]
            n304 = local read "Data File"() -> (w952:path)
            n305 = call "Recorded Values.vi"("Path"=w952) -> ("Recorded Char"=w954:T5, "Recorded Prop"=w955:T6, "Fabrication Prop"=w953:T7)  [unwired: 8 in]
            n306 = Unbundle By Name(w954) -> ("Mobility-Sat"=w968:dbl, "Moblitity-Lin"=w969:dbl, "On/Off"=w970:dbl, "Threshold Voltage"=w971:dbl, "STS"=w972:dbl, "Trap Density-VT"=w973:dbl, "Trap Density-STS"=w974:dbl)  [unwired: 1 out]
            n307 = Unbundle By Name(w953) -> ("Date Created"=w975:string, "Material"=w956:string, "Solvent"=w957:string, "Concentration"=w958:dbl, "Method"=w959:string, "Dielectric (nm)"=w960:dbl, "Treatment"=w961:string, "Comments"=w962:string)
            n308 = Unbundle By Name(w955) -> ("Date Recorded"=w963:string, "Index"=w964:string, "Length"=w965:dbl, "Width"=w966:dbl, "Sample Temp"=w967:dbl)
            n309 = local write "Date Created"(w975) -> ()
            n310 = local write "Rec: VT-Sat"(w971) -> ()
            n311 = local write "Rec: Material"(w956) -> ()
            n312 = local write "Rec: Concentration"(w958) -> ()
            n313 = local write "Rec: Method"(w959) -> ()
            n314 = local write "Rec: Dielectric (d)"(w960) -> ()
            n315 = local write "Surface Treatment:"(w961) -> ()
            n316 = local write "Comments"(w962) -> ()
            n317 = local write "Index"(w964) -> ()
            n318 = local write "Rec: Mobility-Sat"(w968) -> ()
            n319 = local write "Rec: Mobility-Lin"(w969) -> ()
            n320 = local write "Rec: On/Off"(w970) -> ()
            n321 = local write "Rec: STS"(w972) -> ()
            n322 = local write "Rec: Trap Density-VT"(w973) -> ()
            n323 = local write "Rec: Trap Density-STS"(w974) -> ()
            n324 = local write "Rec: Solvent"(w957) -> ()
            n325 = local write "Date Recorded"(w963) -> ()
            n326 = local write "Rec: Length"(w965) -> ()
            n327 = local write "Rec: Width"(w966) -> ()
            n328 = local write "Rec: Temp"(w967) -> ()
            n329 = local read "Data File"() -> (w941:path)
            n330 = Strip Path(path=w941) -> (stripped path=w932:path, name=w950:string)
            n331 = local write "Data Folder"(w932) -> ()
            n332 = List Folder(path=w932) -> (filenames=w946:string[], error out=w886:errorcluster)  [unwired: 3 in, 2 out]
            n333 = local read "Folder Index"() -> (w888:dbl)
            n334 = property on="Image Out" class="ImageControl"() -> (error out=w889:errorcluster, "Image Center Position"=w893:cluster{"X":u32, "Y":u32})  [unwired: 2 in, 1 out]
            n335 = Array Size(array=w946) -> (size(s)=w942:i32)
            n336 = Search 1D Array(1D array=w946, element=w950) -> (index of element=w943:i32)  [unwired: 1 in]
            n337 = Decrement(x=w942) -> (x-1=w944:i32)
            n338 = Equal?(x=w943, y=w944) -> (x = y?=w945:bool)
            n339 = invoke on="Image Out" class="ImageControl" method="Clear ROI"() -> ()  [unwired: 3 in, 3 out]
            n340 = case shown="False" w945 {
              tunnel: w888 -> [w1103 _]
              tunnel: [w1102 0] -> w887
              tunnel: w886 -> [w1101 w1104]
              tunnel: [w1101 w1104] -> w885
              frame False {
                n341 = Increment(x=w1103) -> (x+1=w1102:dbl)
              }
              frame True {
              }
            }
            n342 = Unbundle(w893) -> ("X"=w891:u32)  [unwired: 1 out]
            n343 = local write "Folder Index"(w887) -> ()
            n344 = Bundle("X"=w891, 0) -> (w892:cluster{"X":u32, i32})  [unwired: 1 in]
            n345 = property on="Image Out" class="ImageControl"(error in=w889, "Image Center Position"=w892) -> ()  [unwired: 1 in, 2 out]
            n346 = Path To String(path=w932) -> (string=w951:string)
            n347 = Index Array(array=w946, index=w887) -> (element=w947:string)
            n348 = local write "Data Name:"(w947) -> ()
            n349 = Concatenate Strings(w951, "\\", w947) -> (w949:string)
            n350 = String To Path(string=w949) -> (path=w884:path)
            n351 = local read "NumPts 2"() -> (w879:dbl)
            n352 = local read "NumPts"() -> (w883:dbl)
            n353 = local write "Data File"(w884) -> ()
            n354 = call-poly <vilib>:"Read From Spreadsheet File.vi"("file path (dialog if empty)"=w884) -> ("all rows"=w938:string[][])  [unwired: 6 in, 4 out]
            n355 = call "Mobility-Vt Calculator-File.vi"("NumPts"=w883, "Path"=w884) -> ("XY Graph-Sat"=w881:cluster{dbl[], dbl[]}[], "XY Graph-Lin"=w867:cluster{dbl[], dbl[]}[], "Output"=w882:T8, "Index-Sat"=w880:dbl, "Index-Lin"=w865:dbl)  [unwired: 4 in, 1 out]
            n356 = local read "New: Dielectric"() -> (w862:dbl)
            n357 = call "STS Calculator-File.vi"("NumPts"=w879, "Path"=w884) -> ("STS Index-Sat"=w878:dbl, "XY Graph-Sat"=w877:cluster{dbl[], dbl[]}[], "Ouput"=w876:cluster{"STS-Sat":dbl, "STS-Lin":dbl})  [unwired: 5 in, 2 out]
            n358 = local read "New: Temp"() -> (w859:dbl)
            n359 = Unbundle By Name(w882) -> ("Mobility-Sat"=w875:dbl, "Vt-Sat"=w861:dbl, "Mobility-Lin"=w874:dbl, "Vt-Lin"=w873:dbl, "Off I-Sat"=w856:dbl)
            n360 = Unbundle By Name(w876) -> ("STS-Sat"=w860:dbl)  [unwired: 1 out]
            n361 = local write "Index 2"(w878) -> ()
            n362 = local write "XY Graph 2"(w877) -> ()
            n363 = local write "MobVi Index"(w880) -> ()
            n364 = local write "Slide"(w880) -> ()
            n365 = local write "XY Graph"(w881) -> ()
            n366 = Array Size(array=w938) -> (size(s)=w937:i32[])
            n367 = call "Trap Density_VT.vi"("VT"=w861, "Dielectric"=w862) -> ("Trap Density-VT"=w858:dbl)
            n368 = call "Trap Density_STS.vi"("Temp (T) [K]"=w859, "S.T.S. (S)"=w860, "Dielectric"=w862) -> ("Trap Density (N)"=w857:dbl)  [unwired: 8 in]
            n369 = local write "Calc: Mobility-Sat"(w875) -> ()
            n370 = local write "Calc: STS"(w860) -> ()
            n371 = local write "Calc: Mobility-Lin"(w873) -> ()
            n372 = local write "Calc: VT-Sat"(w861) -> ()
            n373 = local write "Calc: Off I-Sat"(w856) -> ()
            n374 = local write "Calc: VT-Lin"(w874) -> ()
            n375 = local write "Calc: Trap Density-VT"(w858) -> ()
            n376 = local write "Calc: Trap Density-STS"(w857) -> ()
            n377 = local write "New: Trap Density-STS"(w857) -> ()
            n378 = local write "New: Trap Density-VT"(w858) -> ()
            n379 = Index Array(array=w937, index=w936) -> (element=w918:i32)
            n380 = Decimate 1D Array(w877) -> (w912:cluster{dbl[], dbl[]}[])  [unwired: 1 out]
            n381 = Decimate 1D Array(w881) -> (w922:cluster{dbl[], dbl[]}[])  [unwired: 1 out]
            n382 = Decimate 1D Array(w867) -> (w872:cluster{dbl[], dbl[]}[])  [unwired: 1 out]
            n383 = Array Subset(array=w938, index (row)=w936, index (col)=w936, length (col)=3) -> (w939:string[][])  [unwired: 1 in]
            n384 = Array To Cluster(array=w912) -> (cluster=w910:T9)
            n385 = Array To Cluster(array=w922) -> (cluster=w924:T9)
            n386 = Reshape Array(w939, w918) -> (w925:string[])
            n387 = Array To Cluster(array=w872) -> (cluster=w871:T9)
            n388 = Subtract(x=w918, y=20) -> (x-y=w917:i32)
            n389 = local write "New: Mobility-Sat"(w875) -> ()
            n390 = local write "New: Mobility-Lin"(w874) -> ()
            n391 = local write "New: VT-Sat"(w861) -> ()
            n392 = local write "New: VT-Lin"(w873) -> ()
            n393 = property on="Slide" class="Slide (strict)"("Scale.Maximum"=w917) -> ()  [unwired: 2 in, 2 out]
            n394 = Unbundle(w910) -> ("[0]"=w911:cluster{dbl[], dbl[]})  [unwired: 8 out]
            n395 = Unbundle(w924) -> ("[0]"=w923:cluster{dbl[], dbl[]})  [unwired: 8 out]
            n396 = Unbundle(w871) -> ("[0]"=w868:cluster{dbl[], dbl[]})  [unwired: 8 out]
            n397 = Search 1D Array(1D array=w925, element="Index:") -> (index of element=w933:i32)  [unwired: 1 in]
            n398 = local read "NumPts"() -> (w866:dbl)
            n399 = Unbundle(w868) -> (w870:dbl[], w869:dbl[])
            n400 = Increment(x=w933) -> (x+1=w934:i32)
            n401 = Unbundle(w911) -> (w909:dbl[], w908:dbl[])
            n402 = Unbundle(w923) -> (w914:dbl[], w913:dbl[])
            n403 = Array Subset(array=w870, index=w865, length=w866) -> (w864:dbl[])
            n404 = Array Subset(array=w869, index=w865, length=w866) -> (w863:dbl[])
            n405 = Array Subset(array=w909, index=w878, length=w879) -> (w916:dbl[])
            n406 = Array Subset(array=w908, index=w878, length=w879) -> (w915:dbl[])
            n407 = Array Subset(array=w914, index=w880, length=w883) -> (w921:dbl[])
            n408 = Array Subset(array=w913, index=w880, length=w883) -> (w920:dbl[])
            n409 = Index Array(array=w925, index=w934) -> (element=w897:string)
            n410 = local write "Lin-Vg Array-Used"(w864) -> ()
            n411 = local write "Sat Vg Array-Used"(w921) -> ()
            n412 = local write "Vg Array-Log-Used"(w915) -> ()
            n413 = local write "Lin Id-Used"(w863) -> ()
            n414 = local read "Image Folder"() -> (w895:path)
            n415 = local write "Sat Id-Used"(w920) -> ()
            n416 = local write "Sat Id-Log-Used"(w916) -> ()
            n417 = List Folder(path=w895, error in=w885) -> (filenames=w931:string[], error out=w898:errorcluster)  [unwired: 2 in, 2 out]
            n418 = while {
              tunnel: w931 -> [w988]
              tunnel: w897 -> [w986]
              tunnel: [w985] -> _
              tunnel: [w985] -> w930
              tunnel: w918 -> [w984]
              i -> [w985]
              stop <- w981 stop-if-true
              n419 = Index Array(array=w988, index=w985) -> (element=w989:string)
              n420 = xnode "Match Regular Expression"("input string"=w989, "regular expression"=w986) -> ("whole match"=w987:string)  [unwired: 4 in, 4 out]
              n421 = Equal?(x=w987, y=w986) -> (x = y?=w983:bool)
              n422 = Equal?(x=w984, y=w985) -> (x = y?=w982:bool)
              n423 = Or(x=w983, y=w982) -> (x .or. y?=w981:bool)
            }
            n424 = Build Path(base path=w895, name or relative path="ROI") -> (appended path=w894:path)
            n425 = Path To String(path=w895) -> (string=w928:string)
            n426 = Index Array(array=w931, index=w930) -> (element=w906:string)
            n427 = invoke on="Image Out" class="ImageControl" method="Clear ROI"(error in=w898) -> (error out=w901:errorcluster)  [unwired: 2 in, 2 out]
            n428 = local write "Image Name"(w906) -> ()
            n429 = Build Path(base path=w894, name or relative path=w897) -> (appended path=w902:path)
            n430 = call <vilib>:"Check if File or Folder Exists.vi"("error in (no error)"=w901, "path"=w902) -> ("file or folder exists?"=w899:bool, "dup path"=w900:path)  [unwired: 7 in, 1 out]
            n431 = Concatenate Strings(w928, "\\", w906) -> (w927:string)
            n432 = case shown="True" w899 {
              tunnel: w900 -> [_ w976]
              frame False {
              }
              frame True {
                n433 = Read from Text File(file (use dialog)=w976) -> (text=w980:string)  [unwired: 3 in, 3 out]
                n434 = property on="Image Out" class="ImageControl"() -> ("ROI"=w977:T10)  [unwired: 2 in, 2 out]
                n435 = Unflatten From String(type=w977, binary string=w980) -> (value=w978:T10, error out=w979:errorcluster)  [unwired: 3 in, 1 out]
                n436 = property on="Image Out" class="ImageControl"(error in=w979, "ROI"=w978) -> ()  [unwired: 1 in, 2 out]
              }
            }
            n437 = String To Path(string=w927) -> (path=w905:path)
            n438 = Empty String/Path?(string/path=w906) -> (empty?=w907:bool)
            n439 = local read "No Image"() -> (w903:path)
            n440 = Select(t=w903, s=w907, f=w905) -> (s? t:f=w904:path)
            n441 = local write "Image File"(w904) -> ()
            n442 = call "Vision Acquisition4"("Image Path"=w904) -> ("Image Out"=w929:T2)  [unwired: 25 in, 1 out]
            n443 = local write "Image Out"(w929) -> ()
            n444 = local write "Image Out 2"(w929) -> ()
          }
          event "Data File": Value Change {
            w1210 = 0
            n445 = event-data() -> ()  [unwired: 1 in, 5 out]
            n446 = local read "Data File"() -> (w1159:path)
            n447 = call "Recorded Values.vi"("Path"=w1159) -> ("Recorded Char"=w1157:T5, "Recorded Prop"=w1156:T6, "Fabrication Prop"=w1158:T7)  [unwired: 8 in]
            n448 = Unbundle By Name(w1157) -> ("Mobility-Sat"=w1143:dbl, "Moblitity-Lin"=w1142:dbl, "On/Off"=w1141:dbl, "Threshold Voltage"=w1140:dbl, "STS"=w1139:dbl, "Trap Density-VT"=w1138:dbl, "Trap Density-STS"=w1137:dbl)  [unwired: 1 out]
            n449 = Unbundle By Name(w1158) -> ("Date Created"=w1136:string, "Material"=w1155:string, "Solvent"=w1154:string, "Concentration"=w1153:dbl, "Method"=w1152:string, "Dielectric (nm)"=w1151:dbl, "Treatment"=w1150:string, "Comments"=w1149:string)
            n450 = Unbundle By Name(w1156) -> ("Date Recorded"=w1148:string, "Index"=w1147:string, "Length"=w1146:dbl, "Width"=w1145:dbl, "Sample Temp"=w1144:dbl)
            n451 = local write "Date Created"(w1136) -> ()
            n452 = local read "Data File"() -> (w1206:path)
            n453 = local write "Rec: Material"(w1155) -> ()
            n454 = local write "Rec: VT-Sat"(w1140) -> ()
            n455 = local write "Rec: Concentration"(w1153) -> ()
            n456 = local write "Rec: Method"(w1152) -> ()
            n457 = local write "Rec: Dielectric (d)"(w1151) -> ()
            n458 = local write "Surface Treatment:"(w1150) -> ()
            n459 = local write "Comments"(w1149) -> ()
            n460 = local write "Index"(w1147) -> ()
            n461 = local write "Rec: Mobility-Sat"(w1143) -> ()
            n462 = local write "Rec: Mobility-Lin"(w1142) -> ()
            n463 = local write "Rec: On/Off"(w1141) -> ()
            n464 = local write "Rec: STS"(w1139) -> ()
            n465 = local write "Rec: Trap Density-VT"(w1138) -> ()
            n466 = local write "Rec: Trap Density-STS"(w1137) -> ()
            n467 = Strip Path(path=w1206) -> (stripped path=w1205:path, name=w1219:string)
            n468 = local write "Rec: Solvent"(w1154) -> ()
            n469 = local write "Date Recorded"(w1148) -> ()
            n470 = local write "Rec: Length"(w1146) -> ()
            n471 = local write "Rec: Width"(w1145) -> ()
            n472 = local write "Rec: Temp"(w1144) -> ()
            n473 = local write "Data Folder"(w1205) -> ()
            n474 = property on="Image Out" class="ImageControl"() -> (error out=w1161:errorcluster, "Image Center Position"=w1165:cluster{"X":u32, "Y":u32})  [unwired: 2 in, 1 out]
            n475 = List Folder(path=w1205) -> (filenames=w1215:string[], error out=w1171:errorcluster)  [unwired: 3 in, 2 out]
            n476 = Search 1D Array(1D array=w1215, element=w1219) -> (index of element=w1160:i32)  [unwired: 1 in]
            n477 = local write "Folder Index"(w1160) -> ()
            n478 = Unbundle(w1165) -> ("X"=w1163:u32)  [unwired: 1 out]
            n479 = Path To String(path=w1205) -> (string=w1220:string)
            n480 = Index Array(array=w1215, index=w1160) -> (element=w1216:string)
            n481 = Bundle("X"=w1163, 0) -> (w1164:cluster{"X":u32, i32})  [unwired: 1 in]
            n482 = local write "Data Name:"(w1216) -> ()
            n483 = property on="Image Out" class="ImageControl"(error in=w1161, "Image Center Position"=w1164) -> ()  [unwired: 1 in, 2 out]
            n484 = Concatenate Strings(w1220, "\\", w1216) -> (w1218:string)
            n485 = String To Path(string=w1218) -> (path=w1135:path)
            n486 = local read "NumPts 2"() -> (w1130:dbl)
            n487 = local write "Data File"(w1135) -> ()
            n488 = local read "NumPts"() -> (w1131:dbl)
            n489 = local read "New: Dielectric"() -> (w1112:dbl)
            n490 = local read "New: Temp"() -> (w1111:dbl)
            n491 = call-poly <vilib>:"Read From Spreadsheet File.vi"("file path (dialog if empty)"=w1135) -> ("all rows"=w1212:string[][])  [unwired: 6 in, 4 out]
            n492 = call "STS Calculator-File.vi"("NumPts"=w1130, "Path"=w1135) -> ("STS Index-Sat"=w1128:dbl, "XY Graph-Sat"=w1129:cluster{dbl[], dbl[]}[], "Ouput"=w1127:cluster{"STS-Sat":dbl, "STS-Lin":dbl})  [unwired: 5 in, 2 out]
            n493 = call "Mobility-Vt Calculator-File.vi"("NumPts"=w1131, "Path"=w1135) -> ("XY Graph-Sat"=w1134:cluster{dbl[], dbl[]}[], "XY Graph-Lin"=w1124:cluster{dbl[], dbl[]}[], "Output"=w1132:T8, "Index-Sat"=w1133:dbl, "Index-Lin"=w1119:dbl)  [unwired: 4 in, 1 out]
            n494 = Unbundle By Name(w1132) -> ("Mobility-Sat"=w1115:dbl, "Vt-Sat"=w1107:dbl, "Mobility-Lin"=w1114:dbl, "Mobility-Lin"=w1113:dbl, "Off I-Sat"=w1106:dbl)
            n495 = local write "Index 2"(w1128) -> ()
            n496 = local write "XY Graph 2"(w1129) -> ()
            n497 = Unbundle By Name(w1127) -> ("STS-Sat"=w1108:dbl)  [unwired: 1 out]
            n498 = local write "MobVi Index"(w1133) -> ()
            n499 = Array Size(array=w1212) -> (size(s)=w1211:i32[])
            n500 = call "Trap Density_VT.vi"("VT"=w1107, "Dielectric"=w1112) -> ("Trap Density-VT"=w1110:dbl)
            n501 = call "Trap Density_STS.vi"("Temp (T) [K]"=w1111, "S.T.S. (S)"=w1108, "Dielectric"=w1112) -> ("Trap Density (N)"=w1109:dbl)  [unwired: 8 in]
            n502 = local write "Slide"(w1133) -> ()
            n503 = local write "Calc: Mobility-Sat"(w1115) -> ()
            n504 = local write "Calc: Mobility-Lin"(w1113) -> ()
            n505 = local write "Calc: Off I-Sat"(w1106) -> ()
            n506 = local write "Calc: VT-Sat"(w1107) -> ()
            n507 = local write "Calc: VT-Lin"(w1114) -> ()
            n508 = local write "Calc: STS"(w1108) -> ()
            n509 = local write "Calc: Trap Density-VT"(w1110) -> ()
            n510 = local write "Calc: Trap Density-STS"(w1109) -> ()
            n511 = local write "New: Trap Density-STS"(w1109) -> ()
            n512 = local write "New: Trap Density-VT"(w1110) -> ()
            n513 = Decimate 1D Array(w1124) -> (w1126:cluster{dbl[], dbl[]}[])  [unwired: 1 out]
            n514 = Decimate 1D Array(w1129) -> (w1186:cluster{dbl[], dbl[]}[])  [unwired: 1 out]
            n515 = Index Array(array=w1211, index=w1210) -> (element=w1192:i32)
            n516 = Decimate 1D Array(w1134) -> (w1195:cluster{dbl[], dbl[]}[])  [unwired: 1 out]
            n517 = local write "XY Graph"(w1134) -> ()
            n518 = Array Subset(array=w1212, index (row)=w1210, index (col)=w1210, length (col)=3) -> (w1213:string[][])  [unwired: 1 in]
            n519 = Array To Cluster(array=w1126) -> (cluster=w1125:T9)
            n520 = local write "New: STS"(w1108) -> ()
            n521 = Array To Cluster(array=w1186) -> (cluster=w1184:T9)
            n522 = Array To Cluster(array=w1195) -> (cluster=w1197:T9)
            n523 = Reshape Array(w1213, w1192) -> (w1198:string[])
            n524 = local write "New: Mobility-Sat"(w1115) -> ()
            n525 = local write "New: Mobility-Lin"(w1114) -> ()
            n526 = Subtract(x=w1192, y=20) -> (x-y=w1190:i32)
            n527 = local write "New: VT-Sat"(w1107) -> ()
            n528 = local write "New: VT-Lin"(w1113) -> ()
            n529 = Unbundle(w1125) -> ("[0]"=w1123:cluster{dbl[], dbl[]})  [unwired: 8 out]
            n530 = property on="Slide" class="Slide (strict)"("Scale.Maximum"=w1190) -> ()  [unwired: 2 in, 2 out]
            n531 = local read "NumPts"() -> (w1120:dbl)
            n532 = Unbundle(w1123) -> (w1122:dbl[], w1121:dbl[])
            n533 = Unbundle(w1184) -> ("[0]"=w1185:cluster{dbl[], dbl[]})  [unwired: 8 out]
            n534 = Unbundle(w1197) -> ("[0]"=w1196:cluster{dbl[], dbl[]})  [unwired: 8 out]
            n535 = Search 1D Array(1D array=w1198, element="Index:") -> (index of element=w1207:i32)  [unwired: 1 in]
            n536 = local read "NumPts"() -> (w1116:dbl)
            n537 = Array Subset(array=w1122, index=w1119, length=w1120) -> (w1118:dbl[])
            n538 = Array Subset(array=w1121, index=w1119, length=w1120) -> (w1117:dbl[])
            n539 = Increment(x=w1207) -> (x+1=w1208:i32)
            n540 = Unbundle(w1185) -> (w1182:dbl[], w1181:dbl[])
            n541 = Unbundle(w1196) -> (w1183:dbl[], w1187:dbl[])
            n542 = local read "Image Folder"() -> (w1167:path)
            n543 = local write "Lin-Vg Array-Used"(w1118) -> ()
            n544 = Array Subset(array=w1182, index=w1128, length=w1130) -> (w1189:dbl[])
            n545 = Array Subset(array=w1181, index=w1128, length=w1130) -> (w1188:dbl[])
            n546 = Array Subset(array=w1183, index=w1133, length=w1116) -> (w1194:dbl[])
            n547 = Array Subset(array=w1187, index=w1133, length=w1116) -> (w1193:dbl[])
            n548 = Index Array(array=w1198, index=w1208) -> (element=w1169:string)
            n549 = local write "Lin Id-Used"(w1117) -> ()
            n550 = local write "Sat Vg Array-Used"(w1194) -> ()
            n551 = local write "Vg Array-Log-Used"(w1188) -> ()
            n552 = local write "Sat Id-Log-Used"(w1189) -> ()
            n553 = local write "Sat Id-Used"(w1193) -> ()
            n554 = local write "Index"(w1169) -> ()
            n555 = List Folder(path=w1167, error in=w1171) -> (filenames=w1203:string[], error out=w1170:errorcluster)  [unwired: 2 in, 2 out]
            n556 = Build Path(base path=w1167, name or relative path="ROI") -> (appended path=w1166:path)
            n557 = while {
              tunnel: w1203 -> [w1233]
              tunnel: w1169 -> [w1231]
              tunnel: [w1230] -> _
              tunnel: [w1230] -> w1202
              tunnel: w1192 -> [w1229]
              i -> [w1230]
              stop <- w1226 stop-if-true
              n558 = Index Array(array=w1233, index=w1230) -> (element=w1234:string)
              n559 = xnode "Match Regular Expression"("input string"=w1234, "regular expression"=w1231) -> ("whole match"=w1232:string)  [unwired: 4 in, 4 out]
              n560 = Equal?(x=w1232, y=w1231) -> (x = y?=w1228:bool)
              n561 = Equal?(x=w1229, y=w1230) -> (x = y?=w1227:bool)
              n562 = Or(x=w1228, y=w1227) -> (x .or. y?=w1226:bool)
            }
            n563 = invoke on="Image Out" class="ImageControl" method="Clear ROI"(error in=w1170) -> (error out=w1174:errorcluster)  [unwired: 2 in, 2 out]
            n564 = Build Path(base path=w1166, name or relative path=w1169) -> (appended path=w1175:path)
            n565 = call <vilib>:"Check if File or Folder Exists.vi"("error in (no error)"=w1174, "path"=w1175) -> ("file or folder exists?"=w1172:bool, "dup path"=w1173:path)  [unwired: 7 in, 1 out]
            n566 = case shown="True" w1172 {
              tunnel: w1173 -> [_ w1221]
              frame False {
              }
              frame True {
                n567 = Read from Text File(file (use dialog)=w1221) -> (text=w1225:string)  [unwired: 3 in, 3 out]
                n568 = property on="Image Out" class="ImageControl"() -> ("ROI"=w1222:T10)  [unwired: 2 in, 2 out]
                n569 = Unflatten From String(type=w1222, binary string=w1225) -> (value=w1223:T10, error out=w1224:errorcluster)  [unwired: 3 in, 1 out]
                n570 = property on="Image Out" class="ImageControl"(error in=w1224, "ROI"=w1223) -> ()  [unwired: 1 in, 2 out]
              }
            }
            n571 = invoke on="Image Out" class="ImageControl" method="Clear ROI"() -> ()  [unwired: 3 in, 3 out]
            n572 = Path To String(path=w1167) -> (string=w1201:string)
            n573 = Index Array(array=w1203, index=w1202) -> (element=w1179:string)
            n574 = Concatenate Strings(w1201, "\\", w1179) -> (w1200:string)
            n575 = local write "Image Name"(w1179) -> ()
            n576 = String To Path(string=w1200) -> (path=w1178:path)
            n577 = Empty String/Path?(string/path=w1179) -> (empty?=w1180:bool)
            n578 = local read "No Image"() -> (w1176:path)
            n579 = Select(t=w1176, s=w1180, f=w1178) -> (s? t:f=w1177:path)
            n580 = local write "Image File"(w1177) -> ()
            n581 = call "Vision Acquisition3"("Image Path"=w1177) -> ("Image Out"=w1204:T2)  [unwired: 25 in, 1 out]
            n582 = local write "Image Out"(w1204) -> ()
            n583 = local write "Image Out 2"(w1204) -> ()
          }
          event "Up Button": Mouse Down {
            w1451 = 0
            n584 = event-data() -> ()  [unwired: 1 in, 5 out]
            n585 = local read "Data File"() -> (w1398:path)
            n586 = call "Recorded Values.vi"("Path"=w1398) -> ("Recorded Char"=w1396:T5, "Recorded Prop"=w1395:T6, "Fabrication Prop"=w1397:T7)  [unwired: 8 in]
            n587 = Unbundle By Name(w1396) -> ("Mobility-Sat"=w1382:dbl, "Moblitity-Lin"=w1381:dbl, "On/Off"=w1380:dbl, "Threshold Voltage"=w1379:dbl, "STS"=w1378:dbl, "Trap Density-VT"=w1377:dbl, "Trap Density-STS"=w1376:dbl)  [unwired: 1 out]
            n588 = Unbundle By Name(w1397) -> ("Date Created"=w1375:string, "Material"=w1394:string, "Solvent"=w1393:string, "Concentration"=w1392:dbl, "Method"=w1391:string, "Dielectric (nm)"=w1390:dbl, "Treatment"=w1389:string, "Comments"=w1388:string)
            n589 = Unbundle By Name(w1395) -> ("Date Recorded"=w1387:string, "Index"=w1386:string, "Length"=w1385:dbl, "Width"=w1384:dbl, "Sample Temp"=w1383:dbl)
            n590 = local write "Date Created"(w1375) -> ()
            n591 = local write "Rec: Material"(w1394) -> ()
            n592 = local write "Rec: VT-Sat"(w1379) -> ()
            n593 = local write "Rec: Solvent"(w1393) -> ()
            n594 = local write "Rec: Concentration"(w1392) -> ()
            n595 = local write "Rec: Method"(w1391) -> ()
            n596 = local write "Rec: Dielectric (d)"(w1390) -> ()
            n597 = local write "Surface Treatment:"(w1389) -> ()
            n598 = local write "Comments"(w1388) -> ()
            n599 = local write "Index"(w1386) -> ()
            n600 = local write "Rec: Mobility-Sat"(w1382) -> ()
            n601 = local write "Rec: Mobility-Lin"(w1381) -> ()
            n602 = local write "Rec: On/Off"(w1380) -> ()
            n603 = local write "Rec: STS"(w1378) -> ()
            n604 = local write "Rec: Trap Density-VT"(w1377) -> ()
            n605 = local write "Rec: Trap Density-STS"(w1376) -> ()
            n606 = local write "Date Recorded"(w1387) -> ()
            n607 = local write "Rec: Length"(w1385) -> ()
            n608 = local write "Rec: Width"(w1384) -> ()
            n609 = local write "Rec: Temp"(w1383) -> ()
            n610 = local read "Data File"() -> (w1447:path)
            n611 = Strip Path(path=w1447) -> (stripped path=w1446:path, name=w1462:string)
            n612 = local write "Data Folder"(w1446) -> ()
            n613 = List Folder(path=w1446) -> (filenames=w1456:string[], error out=w1413:errorcluster)  [unwired: 3 in, 2 out]
            n614 = Array Size(array=w1456) -> (size(s)=w1401:i32)
            n615 = Search 1D Array(1D array=w1456, element=w1462) -> (index of element=w1457:i32)  [unwired: 1 in]
            n616 = Equal To 0?(x=w1457) -> (x = 0?=w1458:bool)
            n617 = local read "Folder Index"() -> (w1400:dbl)
            n618 = property on="Image Out" class="ImageControl"() -> (error out=w1403:errorcluster, "Image Center Position"=w1407:cluster{"X":u32, "Y":u32})  [unwired: 2 in, 1 out]
            n619 = case shown="True" w1458 {
              tunnel: w1400 -> [w1590 _]
              tunnel: [w1589 w1591] -> w1399
              tunnel: w1401 -> [_ w1592]
              frame False {
                n620 = Decrement(x=w1590) -> (x-1=w1589:dbl)
              }
              frame True {
                n621 = Decrement(x=w1592) -> (x-1=w1591:i32)
              }
            }
            n622 = local write "Folder Index"(w1399) -> ()
            n623 = Unbundle(w1407) -> ("X"=w1405:u32)  [unwired: 1 out]
            n624 = Bundle("X"=w1405, 0) -> (w1406:cluster{"X":u32, i32})  [unwired: 1 in]
            n625 = Path To String(path=w1446) -> (string=w1463:string)
            n626 = Index Array(array=w1456, index=w1399) -> (element=w1459:string)
            n627 = local write "Data Name:"(w1459) -> ()
            n628 = property on="Image Out" class="ImageControl"(error in=w1403, "Image Center Position"=w1406) -> ()  [unwired: 1 in, 2 out]
            n629 = Concatenate Strings(w1463, "\\", w1459) -> (w1461:string)
            n630 = String To Path(string=w1461) -> (path=w1374:path)
            n631 = local read "NumPts 2"() -> (w1369:dbl)
            n632 = local write "Data File"(w1374) -> ()
            n633 = local read "NumPts"() -> (w1373:dbl)
            n634 = local read "New: Dielectric"() -> (w1352:dbl)
            n635 = call "Mobility-Vt Calculator-File.vi"("NumPts"=w1373, "Path"=w1374) -> ("XY Graph-Sat"=w1371:cluster{dbl[], dbl[]}[], "XY Graph-Lin"=w1356:cluster{dbl[], dbl[]}[], "Output"=w1372:T8, "Index-Sat"=w1370:dbl, "Index-Lin"=w1357:dbl)  [unwired: 4 in, 1 out]
            n636 = call "STS Calculator-File.vi"("NumPts"=w1369, "Path"=w1374) -> ("STS Index-Sat"=w1368:dbl, "XY Graph-Sat"=w1367:cluster{dbl[], dbl[]}[], "Ouput"=w1366:cluster{"STS-Sat":dbl, "STS-Lin":dbl})  [unwired: 5 in, 2 out]
            n637 = call-poly <vilib>:"Read From Spreadsheet File.vi"("file path (dialog if empty)"=w1374) -> ("all rows"=w1453:string[][])  [unwired: 6 in, 4 out]
            n638 = local read "New: Temp"() -> (w1351:dbl)
            n639 = Unbundle By Name(w1372) -> ("Mobility-Sat"=w1355:dbl, "Vt-Sat"=w1347:dbl, "Mobility-Lin"=w1354:dbl, "Mobility-Lin"=w1353:dbl, "Off I-Sat"=w1346:dbl)
            n640 = Unbundle By Name(w1366) -> ("STS-Sat"=w1348:dbl)  [unwired: 1 out]
            n641 = local write "Index 2"(w1368) -> ()
            n642 = local write "XY Graph 2"(w1367) -> ()
            n643 = local write "MobVi Index"(w1370) -> ()
            n644 = local write "Slide"(w1370) -> ()
            n645 = local write "XY Graph"(w1371) -> ()
            n646 = Array Size(array=w1453) -> (size(s)=w1452:i32[])
            n647 = local write "Calc: Mobility-Sat"(w1355) -> ()
            n648 = local write "Calc: Mobility-Lin"(w1353) -> ()
            n649 = call "Trap Density_VT.vi"("VT"=w1347, "Dielectric"=w1352) -> ("Trap Density-VT"=w1350:dbl)
            n650 = call "Trap Density_STS.vi"("Temp (T) [K]"=w1351, "S.T.S. (S)"=w1348, "Dielectric"=w1352) -> ("Trap Density (N)"=w1349:dbl)  [unwired: 8 in]
            n651 = local write "Calc: VT-Sat"(w1347) -> ()
            n652 = local write "Calc: Off I-Sat"(w1346) -> ()
            n653 = local write "Calc: VT-Lin"(w1354) -> ()
            n654 = local write "Calc: STS"(w1348) -> ()
            n655 = local write "New: STS"(w1348) -> ()
            n656 = Decimate 1D Array(w1356) -> (w1365:cluster{dbl[], dbl[]}[])  [unwired: 1 out]
            n657 = local write "Calc: Trap Density-VT"(w1350) -> ()
            n658 = local write "Calc: Trap Density-STS"(w1349) -> ()
            n659 = local write "New: Trap Density-STS"(w1349) -> ()
            n660 = local write "New: Trap Density-VT"(w1350) -> ()
            n661 = Decimate 1D Array(w1367) -> (w1430:cluster{dbl[], dbl[]}[])  [unwired: 1 out]
            n662 = Index Array(array=w1452, index=w1451) -> (element=w1436:i32)
            n663 = Decimate 1D Array(w1371) -> (w1440:cluster{dbl[], dbl[]}[])  [unwired: 1 out]
            n664 = Array To Cluster(array=w1365) -> (cluster=w1364:T9)
            n665 = Array Subset(array=w1453, index (row)=w1451, index (col)=w1451, length (col)=3) -> (w1454:string[][])  [unwired: 1 in]
            n666 = local write "New: Mobility-Sat"(w1355) -> ()
            n667 = local write "New: Mobility-Lin"(w1354) -> ()
            n668 = Array To Cluster(array=w1430) -> (cluster=w1428:T9)
            n669 = Array To Cluster(array=w1440) -> (cluster=w1442:T9)
            n670 = Reshape Array(w1454, w1436) -> (w1443:string[])
            n671 = local write "New: VT-Sat"(w1347) -> ()
            n672 = local write "New: VT-Lin"(w1353) -> ()
            n673 = Subtract(x=w1436, y=20) -> (x-y=w1435:i32)
            n674 = Unbundle(w1364) -> ("[0]"=w1361:cluster{dbl[], dbl[]})  [unwired: 8 out]
            n675 = property on="Slide" class="Slide (strict)"("Scale.Maximum"=w1435) -> ()  [unwired: 2 in, 2 out]
            n676 = Unbundle(w1428) -> ("[0]"=w1429:cluster{dbl[], dbl[]})  [unwired: 8 out]
            n677 = Unbundle(w1442) -> ("[0]"=w1441:cluster{dbl[], dbl[]})  [unwired: 8 out]
            n678 = local read "NumPts"() -> (w1358:dbl)
            n679 = Unbundle(w1361) -> (w1360:dbl[], w1359:dbl[])
            n680 = Search 1D Array(1D array=w1443, element="Index:") -> (index of element=w1448:i32)  [unwired: 1 in]
            n681 = Increment(x=w1448) -> (x+1=w1449:i32)
            n682 = Unbundle(w1429) -> (w1427:dbl[], w1426:dbl[])
            n683 = Unbundle(w1441) -> (w1434:dbl[], w1433:dbl[])
            n684 = Array Subset(array=w1360, index=w1357, length=w1358) -> (w1362:dbl[])
            n685 = Array Subset(array=w1359, index=w1357, length=w1358) -> (w1363:dbl[])
            n686 = local read "Image Folder"() -> (w1402:path)
            n687 = local write "Lin-Vg Array-Used"(w1362) -> ()
            n688 = Array Subset(array=w1427, index=w1368, length=w1369) -> (w1432:dbl[])
            n689 = Array Subset(array=w1426, index=w1368, length=w1369) -> (w1431:dbl[])
            n690 = Array Subset(array=w1434, index=w1370, length=w1373) -> (w1439:dbl[])
            n691 = Array Subset(array=w1433, index=w1370, length=w1373) -> (w1438:dbl[])
            n692 = local write "Lin Id-Used"(w1363) -> ()
            n693 = Index Array(array=w1443, index=w1449) -> (element=w1409:string)
            n694 = local write "Sat Vg Array-Used"(w1439) -> ()
            n695 = local write "Vg Array-Log-Used"(w1431) -> ()
            n696 = local write "Sat Id-Log-Used"(w1432) -> ()
            n697 = local write "Sat Id-Used"(w1438) -> ()
            n698 = local write "Index"(w1409) -> ()
            n699 = List Folder(path=w1402, error in=w1413) -> (filenames=w1445:string[], error out=w1412:errorcluster)  [unwired: 2 in, 2 out]
            n700 = Build Path(base path=w1402, name or relative path="ROI") -> (appended path=w1410:path)
            n701 = while {
              tunnel: w1445 -> [w1476]
              tunnel: w1409 -> [w1474]
              tunnel: [w1473] -> w1444
              tunnel: w1436 -> [w1472]
              i -> [w1473]
              stop <- w1469 stop-if-true
              n702 = Index Array(array=w1476, index=w1473) -> (element=w1477:string)
              n703 = xnode "Match Regular Expression"("input string"=w1477, "regular expression"=w1474) -> ("whole match"=w1475:string)  [unwired: 4 in, 4 out]
              n704 = Equal?(x=w1475, y=w1474) -> (x = y?=w1471:bool)
              n705 = Equal?(x=w1472, y=w1473) -> (x = y?=w1470:bool)
              n706 = Or(x=w1471, y=w1470) -> (x .or. y?=w1469:bool)
            }
            n707 = invoke on="Image Out" class="ImageControl" method="Clear ROI"(error in=w1412) -> (error out=w1416:errorcluster)  [unwired: 2 in, 2 out]
            n708 = Build Path(base path=w1410, name or relative path=w1409) -> (appended path=w1408:path)
            n709 = call <vilib>:"Check if File or Folder Exists.vi"("error in (no error)"=w1416, "path"=w1408) -> ("file or folder exists?"=w1414:bool, "dup path"=w1415:path)  [unwired: 7 in, 1 out]
            n710 = case shown="True" w1414 {
              tunnel: w1415 -> [_ w1464]
              frame False {
              }
              frame True {
                n711 = Read from Text File(file (use dialog)=w1464) -> (text=w1468:string)  [unwired: 3 in, 3 out]
                n712 = property on="Image Out" class="ImageControl"() -> ("ROI"=w1465:T10)  [unwired: 2 in, 2 out]
                n713 = Unflatten From String(type=w1465, binary string=w1468) -> (value=w1466:T10, error out=w1467:errorcluster)  [unwired: 3 in, 1 out]
                n714 = property on="Image Out" class="ImageControl"(error in=w1467, "ROI"=w1466) -> ()  [unwired: 1 in, 2 out]
              }
            }
            n715 = Index Array(array=w1445, index=w1444) -> (element=w1418:string)
            n716 = local write "Image Name"(w1418) -> ()
            n717 = Empty String/Path?(string/path=w1418) -> (empty?=w1425:bool)
            n718 = Build Path(base path=w1402, name or relative path=w1418) -> (appended path=w1417:path)
            n719 = local read "No Image"() -> (w1424:path)
            n720 = Select(t=w1424, s=w1425, f=w1417) -> (s? t:f=w1419:path)
            n721 = call <vilib>:"Get File Extension.vi"("file"=w1419) -> ("lowercase file extension"=w1421:string)  [unwired: 7 in, 3 out]
            n722 = local write "Image File"(w1419) -> ()
            n723 = local write "String"(w1421) -> ()
            n724 = Search 1D Array(1D array=string[] ["bmp", "jpeg", "png", "jpg", "gif"], element=w1421) -> (index of element=w1420:i32)  [unwired: 1 in]
            n725 = call "Vision Acquisition5"("Image Path"=w1419) -> ("Image Out"=w1423:T2)  [unwired: 25 in, 1 out]
            n726 = Less Than 0?(x=w1420) -> ()  [unwired: 1 out]
            n727 = local write "Image Out"(w1423) -> ()
            n728 = local write "Image Out 2"(w1423) -> ()
          }
          event "Save Changes? 3": Mouse Down {
            n729 = event-data() -> ()  [unwired: 1 in, 7 out]
            n730 = local read "Image Folder"() -> (w1593:path)
            n731 = Build Path(base path=w1593, name or relative path="ROI") -> (appended path=w1600:path)
            n732 = call <vilib>:"Check if File or Folder Exists.vi"("path"=w1600) -> ("file or folder exists?"=w1602:bool, "dup path"=w1599:path)  [unwired: 8 in, 1 out]
            n733 = case shown="False" w1602 {
              tunnel: w1599 -> [w1604 w1605]
              tunnel: [w1603 w1605] -> w1594
              frame False {
                n734 = Create Folder(path (use dialog)=w1604) -> (created path=w1603:path)  [unwired: 2 in, 2 out]
              }
              frame True {
              }
            }
            n735 = local read "Index"() -> (w1596:string)
            n736 = property on="Image Out" class="ImageControl"() -> ("ROI"=w1598:T10)  [unwired: 2 in, 2 out]
            n737 = Build Path(base path=w1594, name or relative path=w1596) -> (appended path=w1595:path)
            n738 = Flatten To String(anything=w1598) -> (data string=w1597:string)  [unwired: 3 in, 2 out]
            n739 = Write to Text File(file (use dialog)=w1595, text=w1597) -> ()  [unwired: 2 in, 3 out]
          }
          event "Next Button": Mouse Down {
            n740 = event-data() -> ()  [unwired: 1 in, 5 out]
            n741 = local read "XY Graph"() -> (w1618:cluster{dbl[], dbl[]}[])
            n742 = Decimate 1D Array(w1618) -> (w1614:cluster{dbl[], dbl[]}[], w1613:cluster{dbl[], dbl[]}[])
            n743 = Array To Cluster(array=w1614) -> (cluster=w1624:T9)
            n744 = local read "MobVi Index"() -> (w1620:dbl)
            n745 = Unbundle(w1624) -> ("[0]"=w1623:cluster{dbl[], dbl[]})  [unwired: 8 out]
            n746 = local read "NumPts"() -> (w1619:dbl)
            n747 = Unbundle(w1623) -> (w1622:dbl[], w1621:dbl[])
            n748 = local read "New: Dielectric"() -> (w1609:dbl)
            n749 = Increment(x=w1620) -> (x+1=w1615:dbl)
            n750 = local read "New: Length"() -> (w1608:dbl)
            n751 = local read "New: Width"() -> (w1607:dbl)
            n752 = local write "MobVi Index"(w1615) -> ()
            n753 = Array Subset(array=w1622, index=w1615, length=w1619) -> (w1611:dbl[])
            n754 = Array Subset(array=w1621, index=w1615, length=w1619) -> (w1610:dbl[])
            n755 = local write "Sat Vg Array-Used"(w1611) -> ()
            n756 = local write "Sat Id-Used"(w1610) -> ()
            n757 = call "Mobility-Vt-Used Pts_Saturation.vi"("Width"=w1607, "Length"=w1608, "Dielectric (d)"=w1609, "Sat Id Used"=w1610, "Vg Used"=w1611) -> ("Vt"=w1606:dbl, "Mobility"=w1612:dbl)  [unwired: 4 in, 1 out]
            n758 = Bundle(w1611, w1610) -> (w1617:cluster{dbl[], dbl[]})  [unwired: 1 in]
            n759 = Build Array (concatenate)(w1614, w1613, w1617) -> (w1616:cluster{dbl[], dbl[]}[])
            n760 = local write "New: Mobility-Sat"(w1612) -> ()
            n761 = local write "New: VT-Sat"(w1606) -> ()
            n762 = local write "XY Graph"(w1616) -> ()
          }
          event "Next Button 2": Mouse Down {
            n763 = event-data() -> ()  [unwired: 1 in, 7 out]
            n764 = local read "XY Graph 2"() -> (w1633:cluster{dbl[], dbl[]}[])
            n765 = Decimate 1D Array(w1633) -> (w1629:cluster{dbl[], dbl[]}[], w1628:cluster{dbl[], dbl[]}[])
            n766 = Array To Cluster(array=w1629) -> (cluster=w1639:T9)
            n767 = local read "Index 2"() -> (w1635:dbl)
            n768 = Unbundle(w1639) -> ("[0]"=w1638:cluster{dbl[], dbl[]})  [unwired: 8 out]
            n769 = local read "NumPts 2"() -> (w1634:dbl)
            n770 = Unbundle(w1638) -> (w1637:dbl[], w1636:dbl[])
            n771 = Increment(x=w1635) -> (x+1=w1630:dbl)
            n772 = local write "Index 2"(w1630) -> ()
            n773 = Array Subset(array=w1636, index=w1630, length=w1634) -> (w1625:dbl[])
            n774 = Array Subset(array=w1637, index=w1630, length=w1634) -> (w1626:dbl[])
            n775 = call "STS-Used.vi"("Id Used"=w1626, "Vg-Used"=w1625) -> ("STS"=w1627:dbl)  [unwired: 9 in]
            n776 = Bundle(w1626, w1625) -> (w1632:cluster{dbl[], dbl[]})  [unwired: 1 in]
            n777 = local write "Vg Array-Log-Used"(w1625) -> ()
            n778 = local write "Sat Id-Log-Used"(w1626) -> ()
            n779 = local write "New: STS"(w1627) -> ()
            n780 = Build Array (concatenate)(w1629, w1628, w1632) -> (w1631:cluster{dbl[], dbl[]}[])
            n781 = local write "XY Graph 2"(w1631) -> ()
          }
          event "Previous Button 2": Mouse Down {
            n782 = event-data() -> ()  [unwired: 1 in, 7 out]
            n783 = local read "XY Graph 2"() -> (w1649:cluster{dbl[], dbl[]}[])
            n784 = Decimate 1D Array(w1649) -> (w1646:cluster{dbl[], dbl[]}[], w1645:cluster{dbl[], dbl[]}[])
            n785 = Array To Cluster(array=w1646) -> (cluster=w1654:T9)
            n786 = local read "Index 2"() -> (w1642:dbl)
            n787 = Unbundle(w1654) -> ("[0]"=w1653:cluster{dbl[], dbl[]})  [unwired: 8 out]
            n788 = local read "NumPts 2"() -> (w1650:dbl)
            n789 = Unbundle(w1653) -> (w1652:dbl[], w1651:dbl[])
            n790 = Decrement(x=w1642) -> (x-1=w1643:dbl)
            n791 = local write "Index 2"(w1643) -> ()
            n792 = Array Subset(array=w1652, index=w1643, length=w1650) -> (w1640:dbl[])
            n793 = Array Subset(array=w1651, index=w1643, length=w1650) -> (w1641:dbl[])
            n794 = local write "Vg Array-Log-Used"(w1641) -> ()
            n795 = local write "Sat Id-Log-Used"(w1640) -> ()
            n796 = Bundle(w1640, w1641) -> (w1648:cluster{dbl[], dbl[]})  [unwired: 1 in]
            n797 = call "STS-Used.vi"("Id Used"=w1640, "Vg-Used"=w1641) -> ("STS"=w1644:dbl)  [unwired: 9 in]
            n798 = Build Array (concatenate)(w1646, w1645, w1648) -> (w1647:cluster{dbl[], dbl[]}[])
            n799 = local write "New: STS"(w1644) -> ()
            n800 = local write "XY Graph 2"(w1647) -> ()
          }
          event "Previous Button": Mouse Down {
            n801 = event-data() -> ()  [unwired: 1 in, 5 out]
            n802 = local read "XY Graph"() -> (w1668:cluster{dbl[], dbl[]}[])
            n803 = Decimate 1D Array(w1668) -> (w1665:cluster{dbl[], dbl[]}[], w1664:cluster{dbl[], dbl[]}[])
            n804 = Array To Cluster(array=w1665) -> (cluster=w1673:T9)
            n805 = local read "MobVi Index"() -> (w1663:dbl)
            n806 = Unbundle(w1673) -> ("[0]"=w1672:cluster{dbl[], dbl[]})  [unwired: 8 out]
            n807 = local read "NumPts"() -> (w1669:dbl)
            n808 = Unbundle(w1672) -> (w1671:dbl[], w1670:dbl[])
            n809 = Decrement(x=w1663) -> (x-1=w1662:dbl)
            n810 = local read "New: Dielectric"() -> (w1656:dbl)
            n811 = local read "New: Length"() -> (w1657:dbl)
            n812 = local read "New: Width"() -> (w1658:dbl)
            n813 = local write "MobVi Index"(w1662) -> ()
            n814 = Array Subset(array=w1671, index=w1662, length=w1669) -> (w1661:dbl[])
            n815 = Array Subset(array=w1670, index=w1662, length=w1669) -> (w1660:dbl[])
            n816 = local write "Sat Vg Array-Used"(w1661) -> ()
            n817 = local write "Sat Id-Used"(w1660) -> ()
            n818 = call "Mobility-Vt-Used Pts_Linear.vi"("Width"=w1658, "Length"=w1657, "Dielectric (d)"=w1656, "Sat Id Used"=w1660, "Vg Used"=w1661) -> ("Vt"=w1655:dbl, "Mobility"=w1659:dbl)  [unwired: 4 in, 1 out]
            n819 = Bundle(w1661, w1660) -> (w1667:cluster{dbl[], dbl[]})  [unwired: 1 in]
            n820 = local write "New: VT-Sat"(w1655) -> ()
            n821 = Build Array (concatenate)(w1665, w1664, w1667) -> (w1666:cluster{dbl[], dbl[]}[])
            n822 = local write "New: Mobility-Sat"(w1659) -> ()
            n823 = local write "XY Graph"(w1666) -> ()
          }
          event "Slide": Value Change {
            n824 = event-data() -> ()  [unwired: 1 in, 5 out]
            n825 = local read "XY Graph"() -> (w1686:cluster{dbl[], dbl[]}[])
            n826 = Decimate 1D Array(w1686) -> (w1683:cluster{dbl[], dbl[]}[], w1682:cluster{dbl[], dbl[]}[])
            n827 = Array To Cluster(array=w1683) -> (cluster=w1691:T9)
            n828 = Unbundle(w1691) -> ("[0]"=w1690:cluster{dbl[], dbl[]})  [unwired: 8 out]
            n829 = local read "NumPts"() -> (w1687:dbl)
            n830 = local read "Slide"() -> (w1675:dbl)
            n831 = Unbundle(w1690) -> (w1689:dbl[], w1688:dbl[])
            n832 = local read "New: Dielectric"() -> (w1676:dbl)
            n833 = local read "New: Length"() -> (w1677:dbl)
            n834 = local read "New: Width"() -> (w1678:dbl)
            n835 = local write "MobVi Index"(w1675) -> ()
            n836 = Array Subset(array=w1689, index=w1675, length=w1687) -> (w1681:dbl[])
            n837 = Array Subset(array=w1688, index=w1675, length=w1687) -> (w1680:dbl[])
            n838 = local write "Sat Vg Array-Used"(w1681) -> ()
            n839 = local write "Sat Id-Used"(w1680) -> ()
            n840 = call "Mobility-Vt-Used Pts_Linear.vi"("Width"=w1678, "Length"=w1677, "Dielectric (d)"=w1676, "Sat Id Used"=w1680, "Vg Used"=w1681) -> ("Vt"=w1674:dbl, "Mobility"=w1679:dbl)  [unwired: 4 in, 1 out]
            n841 = Bundle(w1681, w1680) -> (w1685:cluster{dbl[], dbl[]})  [unwired: 1 in]
            n842 = local write "New: VT-Sat"(w1674) -> ()
            n843 = Build Array (concatenate)(w1683, w1682, w1685) -> (w1684:cluster{dbl[], dbl[]}[])
            n844 = local write "New: Mobility-Sat"(w1679) -> ()
            n845 = local write "XY Graph"(w1684) -> ()
          }
          event "Slide 2": Value Change {
            n846 = event-data() -> ()  [unwired: 1 in, 5 out]
            n847 = local read "XY Graph 2"() -> (w1700:cluster{dbl[], dbl[]}[])
            n848 = Decimate 1D Array(w1700) -> (w1697:cluster{dbl[], dbl[]}[], w1696:cluster{dbl[], dbl[]}[])
            n849 = Array To Cluster(array=w1697) -> (cluster=w1705:T9)
            n850 = Unbundle(w1705) -> ("[0]"=w1704:cluster{dbl[], dbl[]})  [unwired: 8 out]
            n851 = local read "NumPts 2"() -> (w1701:dbl)
            n852 = local read "Slide 2"() -> (w1695:dbl)
            n853 = Unbundle(w1704) -> (w1703:dbl[], w1702:dbl[])
            n854 = local write "Index 2"(w1695) -> ()
            n855 = Array Subset(array=w1703, index=w1695, length=w1701) -> (w1693:dbl[])
            n856 = Array Subset(array=w1702, index=w1695, length=w1701) -> (w1692:dbl[])
            n857 = local write "Vg Array-Log-Used"(w1692) -> ()
            n858 = local write "Sat Id-Log-Used"(w1693) -> ()
            n859 = call "STS-Used.vi"("Id Used"=w1693, "Vg-Used"=w1692) -> ("STS"=w1694:dbl)  [unwired: 9 in]
            n860 = Bundle(w1693, w1692) -> (w1699:cluster{dbl[], dbl[]})  [unwired: 1 in]
            n861 = local write "New: STS"(w1694) -> ()
            n862 = Build Array (concatenate)(w1697, w1696, w1699) -> (w1698:cluster{dbl[], dbl[]}[])
            n863 = local write "XY Graph 2"(w1698) -> ()
          }
          event "Save Changes?": Mouse Down {
            n864 = event-data() -> ()  [unwired: 1 in, 5 out]
            n865 = flat-sequence {
              tunnel: [w1768] -> w1711
              tunnel: [w1712] -> w1709
              tunnel: [w1712] -> w1708
              tunnel: [w1713] -> w1706
              tunnel: w1711 -> [w1849]
              tunnel: [w1850] -> w1710
              tunnel: w1709 -> [w1850]
              tunnel: w1708 -> [w1848]
              tunnel: [w1846] -> w1707
              tunnel: w1706 -> [w1846]
              tunnel: w1710 -> [w1855]
              tunnel: w1707 -> [w1854]
              frame #0 {
                n866 = local read "Data File"() -> (w1768:path)
                n867 = call-poly <vilib>:"Read From Spreadsheet File.vi"("file path (dialog if empty)"=w1768) -> ("all rows"=w1721:string[][])  [unwired: 6 in, 4 out]
                n868 = flat-sequence {
                  tunnel: [w1803] -> w1766
                  tunnel: w1766 -> [w1820]
                  frame #0 {
                    # "Makes Empty File for Transformer Data"
                    n869 = local read "Data Folder"() -> (w1792:path)
                    n870 = Build Path(base path=w1792, name or relative path="Stats") -> (appended path=w1794:path)
                    n871 = call <vilib>:"Check if File or Folder Exists.vi"("path"=w1794) -> ("file or folder exists?"=w1795:bool, "dup path"=w1796:path)  [unwired: 8 in, 1 out]
                    n872 = case shown="False" w1795 {
                      tunnel: [w1800 w1802] -> w1797
                      tunnel: w1796 -> [w1801 w1802]
                      frame False {
                        n873 = Create Folder(path (use dialog)=w1801) -> (created path=w1800:path)  [unwired: 2 in, 2 out]
                      }
                      frame True {
                      }
                    }
                    n874 = Build Path(base path=w1797, name or relative path="Tranformer Data.txt") -> (appended path=w1799:path)
                    n875 = call-poly <vilib>:"Write To Spreadsheet File.vi"("append to file? (new file:F)"=TRUE, "file path (dialog if empty)"=w1799) -> ()  [unwired: 6 in, 1 out]
                  }
                  frame #1 {
                    # "Adds Headers if they don't exist"
                    n876 = Concatenate Strings("Stats\\", "Tranformer Data.txt") -> (w1810:string)
                    n877 = local read "Data Folder"() -> (w1809:path)
                    n878 = Build Path(base path=w1809, name or relative path=w1810) -> (appended path=w1803:path)
                    n879 = call-poly <vilib>:"Read From Spreadsheet File.vi"("file path (dialog if empty)"=w1803) -> ("first row"=w1808:string[])  [unwired: 6 in, 4 out]
                    n880 = Search 1D Array(1D array=w1808, element="DeviceID") -> (index of element=w1806:i32)  [unwired: 1 in]
                    n881 = Equal?(x=w1806, y=0) -> (x = y?=w1804:bool)
                    n882 = case shown="False" w1804 {
                      tunnel: w1803 -> [w1814 _]
                      frame False {
                        n883 = local read "Transformer \nHeaders"() -> (w1813:string[])
                        n884 = call-poly <vilib>:"Write To Spreadsheet File.vi"("1D data"=w1813, "file path (dialog if empty)"=w1814) -> ()  [unwired: 6 in, 1 out]
                      }
                      frame True {
                      }
                    }
                  }
                  frame #2 {
                    # "Adds current device if it doesn't exist"
                    n885 = local read "Current \nRecord"() -> (w1819:string[])
                    n886 = Index Array(array=w1819, index=0) -> (element=w1818:string)
                    n887 = Concatenate Strings("Stats\\", "Tranformer Data.txt") -> (w1823:string)
                    n888 = local read "Data Folder"() -> (w1822:path)
                    n889 = local write "Current Device ID"(w1818) -> ()
                    n890 = local read "Current Device ID"() -> (w1828:string)
                    n891 = Build Path(base path=w1822, name or relative path=w1823) -> (appended path=w1821:path)
                    n892 = call-poly <vilib>:"Read From Spreadsheet File.vi"("file path (dialog if empty)"=w1821) -> ("all rows"=w1815:string[][])  [unwired: 6 in, 4 out]
                    n893 = Index Array(array=w1815, index (col)=0) -> (element=w1816:string[])  [unwired: 1 in]
                    n894 = Search 1D Array(1D array=w1816, element=w1828) -> (index of element=w1817:i32)  [unwired: 1 in]
                    n895 = Equal?(x=w1817, y=-1) -> (x = y?=w1830:bool)
                    n896 = case shown="False" w1830 {
                      tunnel: w1820 -> [w1833 w1844]
                      tunnel: w1817 -> [w1836 _]
                      tunnel: w1815 -> [w1837 _]
                      frame False {
                        n897 = local read "Current \nRecord"() -> (w1835:string[])
                        n898 = Replace Array Subset(array=w1837, new element=w1835, index (row)=w1836) -> (w1834:string[][])  [unwired: 1 in]
                        n899 = flat-sequence {
                          tunnel: w1833 -> [w1838]
                          tunnel: w1834 -> [w1839]
                          tunnel: [w1839] -> w1832
                          tunnel: [w1838] -> w1831
                          tunnel: w1832 -> [w1841]
                          tunnel: w1831 -> [w1840]
                          frame #0 {
                            n900 = Delete(path (use dialog)=w1838) -> ()  [unwired: 4 in, 3 out]
                          }
                          frame #1 {
                            n901 = call-poly <vilib>:"Write To Spreadsheet File.vi"("append to file? (new file:F)"=TRUE, "2D data"=w1841, "file path (dialog if empty)"=w1840) -> ()  [unwired: 5 in, 1 out]
                          }
                        }
                      }
                      frame True {
                        n902 = local read "Current \nRecord"() -> (w1843:string[])
                        n903 = call-poly <vilib>:"Write To Spreadsheet File.vi"("append to file? (new file:F)"=TRUE, "1D data"=w1843, "file path (dialog if empty)"=w1844) -> ()  [unwired: 5 in, 1 out]
                      }
                    }
                  }
                }
                n904 = local read "New: Dielectric"() -> (w1759:dbl)
                n905 = local read "New: Mobility-Sat"() -> (w1751:dbl)
                n906 = Number To Fractional String(number=w1759) -> (F-format string=w1771:string)  [unwired: 3 in]
                n907 = local read "New: Temp"() -> (w1762:dbl)
                n908 = local read "New: STS"() -> (w1724:dbl)
                n909 = Number To Fractional String(number=w1751) -> (F-format string=w1747:string)  [unwired: 3 in]
                n910 = Number To Fractional String(number=w1724) -> (F-format string=w1727:string)  [unwired: 3 in]
                n911 = local read "New: Length"() -> (w1758:dbl)
                n912 = Replace Array Subset(array=w1721, new element=w1771, index (row)=7, index (col)=1) -> (w1775:string[][])
                n913 = local read "New: Width"() -> (w1760:dbl)
                n914 = local read "New: Length"() -> (w1780:dbl)
                n915 = Number To Decimal String(number=w1762) -> (decimal integer string=w1764:string)  [unwired: 1 in]
                n916 = local read "New: Trap Density-VT"() -> (w1732:dbl)
                n917 = local read "New: Mobility-Lin"() -> (w1740:dbl)
                n918 = Number To Fractional String(number=w1780) -> (F-format string=w1781:string)  [unwired: 3 in]
                n919 = Number To Fractional String(number=w1740) -> (F-format string=w1739:string)  [unwired: 3 in]
                n920 = Number To Fractional String(number=w1732) -> (F-format string=w1733:string)  [unwired: 3 in]
                n921 = local read "Index"() -> (w1783:string)
                n922 = Strip Path(path=w1768) -> (stripped path=w1788:path)  [unwired: 1 out]
                n923 = Number To Decimal String(number=w1758) -> (decimal integer string=w1778:string)  [unwired: 1 in]
                n924 = Number To Decimal String(number=w1760) -> (decimal integer string=w1779:string)  [unwired: 1 in]
                n925 = Concatenate Strings("_", w1764, "K") -> (w1761:string)
                n926 = Replace Array Subset(array=w1775, new element=w1781, index (row)=12, index (col)=1) -> (w1777:string[][])
                n927 = call "Build Text"("Temp"=w1761, "Index"=w1783, "Length"=w1778, "Width"=w1779) -> ("Result"=w1784:string)  [unwired: 10 in, 1 out]
                n928 = local read "New: Width"() -> (w1789:dbl)
                n929 = local read "New: VT-Sat"() -> (w1737:dbl)
                n930 = Number To Fractional String(number=w1789) -> (F-format string=w1769:string)  [unwired: 3 in]
                n931 = local read "New: Trap Density-VT"() -> (w1735:dbl)
                n932 = Number To Fractional String(number=w1737) -> (F-format string=w1749:string)  [unwired: 3 in]
                n933 = Number To Fractional String(number=w1735) -> (F-format string=w1726:string)  [unwired: 3 in]
                n934 = Path To String(path=w1788) -> (string=w1786:string)
                n935 = Replace Array Subset(array=w1777, new element=w1769, index (row)=13, index (col)=1) -> (w1776:string[][])
                n936 = local read "Calc: Off I-Sat"() -> (w1718:dbl)
                n937 = Concatenate Strings(w1786, "\\", w1784) -> (w1785:string)
                n938 = local read "New: Temp"() -> (w1790:dbl)
                n939 = Number To Fractional String(number=w1790) -> (F-format string=w1770:string)  [unwired: 3 in]
                n940 = local read "New: VT-Lin"() -> (w1736:dbl)
                n941 = Number To Fractional String(number=w1736) -> (F-format string=w1748:string)  [unwired: 3 in]
                n942 = String To Path(string=w1785) -> (path=w1712:path)
                n943 = Number To Fractional String(number=w1718) -> (F-format string=w1714:string)  [unwired: 3 in]
                n944 = Replace Array Subset(array=w1776, new element=w1770, index (row)=14, index (col)=1) -> (w1720:string[][])
                n945 = Replace Array Subset(array=w1720, new element=w1747, index (row)=16, index (col)=1) -> (w1743:string[][])
                n946 = Replace Array Subset(array=w1743, new element=w1739, index (row)=17, index (col)=1) -> (w1741:string[][])
                n947 = Replace Array Subset(array=w1741, new element=w1749, index (row)=19, index (col)=1) -> (w1742:string[][])
                n948 = Replace Array Subset(array=w1742, new element=w1748, index (row)=20, index (col)=1) -> (w1719:string[][])
                n949 = Replace Array Subset(array=w1719, new element=w1727, index (row)=21, index (col)=1) -> (w1730:string[][])
                n950 = Replace Array Subset(array=w1730, new element=w1733, index (row)=22, index (col)=1) -> (w1731:string[][])
                n951 = Replace Array Subset(array=w1731, new element=w1726, index (row)=23, index (col)=1) -> (w1717:string[][])
                n952 = Replace Array Subset(array=w1717, new element=w1714, index (row)=0, index (col)=1) -> (w1713:string[][])
              }
              frame #1 {
                n953 = Equal?(x=w1849, y=w1848) -> (x = y?=w1847:bool)
                n954 = case shown="False" w1847 {
                  tunnel: w1849 -> [w1853 _]
                  tunnel: w1848 -> [w1852 _]
                  frame False {
                    n955 = Move(source path=w1853, 9:TRUE, 10:w1852) -> ()  [unwired: 2 in, 3 out]
                  }
                  frame True {
                  }
                }
              }
              frame #2 {
                n956 = local write "Data File"(w1855) -> ()
                n957 = call-poly <vilib>:"Write To Spreadsheet File.vi"("2D data"=w1854, "file path (dialog if empty)"=w1855) -> ()  [unwired: 6 in, 1 out]
              }
            }
          }
          event "Save Changes? 2": Mouse Down {
            n958 = event-data() -> ()  [unwired: 1 in, 5 out]
            n959 = local read "Data File"() -> (w1879:path)
            n960 = call "Recorded Values.vi"("Path"=w1879) -> ("Recorded Char"=w1877:T5, "Recorded Prop"=w1876:T6, "Fabrication Prop"=w1878:T7)  [unwired: 8 in]
            n961 = Unbundle By Name(w1877) -> ("Mobility-Sat"=w1863:dbl, "Moblitity-Lin"=w1862:dbl, "On/Off"=w1861:dbl, "Threshold Voltage"=w1860:dbl, "STS"=w1859:dbl, "Trap Density-VT"=w1858:dbl, "Trap Density-STS"=w1857:dbl)  [unwired: 1 out]
            n962 = Unbundle By Name(w1876) -> ("Date Recorded"=w1868:string, "Index"=w1867:string, "Length"=w1866:dbl, "Width"=w1865:dbl, "Sample Temp"=w1864:dbl)
            n963 = Unbundle By Name(w1878) -> ("Date Created"=w1856:string, "Material"=w1875:string, "Solvent"=w1874:string, "Concentration"=w1873:dbl, "Method"=w1872:string, "Dielectric (nm)"=w1871:dbl, "Treatment"=w1870:string, "Comments"=w1869:string)
            n964 = local write "Rec: VT-Sat"(w1860) -> ()
            n965 = local write "Date Created"(w1856) -> ()
            n966 = local write "Rec: Material"(w1875) -> ()
            n967 = local write "Rec: Solvent"(w1874) -> ()
            n968 = local write "Rec: Concentration"(w1873) -> ()
            n969 = local write "Rec: Method"(w1872) -> ()
            n970 = local write "Rec: Dielectric (d)"(w1871) -> ()
            n971 = local write "Surface Treatment:"(w1870) -> ()
            n972 = local write "Comments"(w1869) -> ()
            n973 = local write "Index"(w1867) -> ()
            n974 = local write "Rec: Mobility-Sat"(w1863) -> ()
            n975 = local write "Rec: Mobility-Lin"(w1862) -> ()
            n976 = local write "Rec: On/Off"(w1861) -> ()
            n977 = local write "Rec: STS"(w1859) -> ()
            n978 = local write "Rec: Trap Density-VT"(w1858) -> ()
            n979 = local write "Rec: Trap Density-STS"(w1857) -> ()
            n980 = local write "Date Recorded"(w1868) -> ()
            n981 = local write "Rec: Length"(w1866) -> ()
            n982 = local write "Rec: Width"(w1865) -> ()
            n983 = local write "Rec: Temp"(w1864) -> ()
            n984 = stacked-sequence {
              seq-local: [w1943 _ _ _ _] -> [_ w2017 _ _ _]
              seq-local: [w1942 _ _ _ _] -> [_ w2018 _ _ _]
              seq-local: [w1943 _ _ _ _] -> [_ w2016 _ _ _]
              seq-local: [w1936 _ _ _ _] -> [_ w2014 _ _ _]
              seq-local: [_ w2018 _ _ _] -> [_ _ w2023 _ _]
              seq-local: [_ w2014 _ _ _] -> [_ _ w2022 _ _]
              frame #0 {
                n985 = local read "Data File"() -> (w1942:path)
                n986 = call-poly <vilib>:"Read From Spreadsheet File.vi"("file path (dialog if empty)"=w1942) -> ("all rows"=w1946:string[][])  [unwired: 6 in, 4 out]
                n987 = local read "New: Dielectric"() -> (w1984:dbl)
                n988 = local read "New: Mobility-Sat"() -> (w1976:dbl)
                n989 = Number To Fractional String(number=w1984) -> (F-format string=w1994:string)  [unwired: 3 in]
                n990 = local read "New: Temp"() -> (w1987:dbl)
                n991 = local read "New: STS"() -> (w1949:dbl)
                n992 = Number To Fractional String(number=w1976) -> (F-format string=w1972:string)  [unwired: 3 in]
                n993 = Number To Fractional String(number=w1949) -> (F-format string=w1952:string)  [unwired: 3 in]
                n994 = local read "New: Length"() -> (w1983:dbl)
                n995 = Replace Array Subset(array=w1946, new element=w1994, index (row)=7, index (col)=1) -> (w1998:string[][])
                n996 = local read "New: Width"() -> (w1985:dbl)
                n997 = local read "New: Length"() -> (w2003:dbl)
                n998 = Number To Decimal String(number=w1987) -> (decimal integer string=w1989:string)  [unwired: 1 in]
                n999 = local read "New: Trap Density-VT"() -> (w1957:dbl)
                n1000 = local read "New: Mobility-Lin"() -> (w1965:dbl)
                n1001 = Number To Fractional String(number=w2003) -> (F-format string=w2004:string)  [unwired: 3 in]
                n1002 = Number To Fractional String(number=w1965) -> (F-format string=w1964:string)  [unwired: 3 in]
                n1003 = Number To Fractional String(number=w1957) -> (F-format string=w1958:string)  [unwired: 3 in]
                n1004 = local read "Index"() -> (w2006:string)
                n1005 = Strip Path(path=w1942) -> (stripped path=w2011:path)  [unwired: 1 out]
                n1006 = Number To Decimal String(number=w1983) -> (decimal integer string=w2001:string)  [unwired: 1 in]
                n1007 = Number To Decimal String(number=w1985) -> (decimal integer string=w2002:string)  [unwired: 1 in]
                n1008 = Concatenate Strings("_", w1989, "K") -> (w1986:string)
                n1009 = Replace Array Subset(array=w1998, new element=w2004, index (row)=12, index (col)=1) -> (w2000:string[][])
                n1010 = call "Build Text3"("Temp"=w1986, "Index"=w2006, "Length"=w2001, "Width"=w2002) -> ("Result"=w2007:string)  [unwired: 10 in, 1 out]
                n1011 = local read "New: Width"() -> (w2012:dbl)
                n1012 = local read "New: VT-Sat"() -> (w1962:dbl)
                n1013 = Number To Fractional String(number=w2012) -> (F-format string=w1992:string)  [unwired: 3 in]
                n1014 = local read "New: Trap Density-VT"() -> (w1960:dbl)
                n1015 = Number To Fractional String(number=w1962) -> (F-format string=w1974:string)  [unwired: 3 in]
                n1016 = Number To Fractional String(number=w1960) -> (F-format string=w1951:string)  [unwired: 3 in]
                n1017 = Path To String(path=w2011) -> (string=w2009:string)
                n1018 = Replace Array Subset(array=w2000, new element=w1992, index (row)=13, index (col)=1) -> (w1999:string[][])
                n1019 = Concatenate Strings(w2009, "\\", w2007) -> (w2008:string)
                n1020 = local read "New: Temp"() -> (w2013:dbl)
                n1021 = Number To Fractional String(number=w2013) -> (F-format string=w1993:string)  [unwired: 3 in]
                n1022 = local read "New: VT-Lin"() -> (w1961:dbl)
                n1023 = local read "Calc: Mobility-Sat"() -> (w1938:dbl)
                n1024 = Number To Fractional String(number=w1961) -> (F-format string=w1973:string)  [unwired: 3 in]
                n1025 = Number To Fractional String(number=w1938) -> (F-format string=w1940:string)  [unwired: 3 in]
                n1026 = String To Path(string=w2008) -> (path=w1943:path)
                n1027 = Replace Array Subset(array=w1999, new element=w1993, index (row)=14, index (col)=1) -> (w1945:string[][])
                n1028 = Replace Array Subset(array=w1945, new element=w1972, index (row)=16, index (col)=1) -> (w1968:string[][])
                n1029 = Replace Array Subset(array=w1968, new element=w1964, index (row)=17, index (col)=1) -> (w1966:string[][])
                n1030 = Replace Array Subset(array=w1966, new element=w1974, index (row)=19, index (col)=1) -> (w1967:string[][])
                n1031 = Replace Array Subset(array=w1967, new element=w1973, index (row)=20, index (col)=1) -> (w1944:string[][])
                n1032 = Replace Array Subset(array=w1944, new element=w1952, index (row)=21, index (col)=1) -> (w1955:string[][])
                n1033 = Replace Array Subset(array=w1955, new element=w1958, index (row)=22, index (col)=1) -> (w1956:string[][])
                n1034 = Replace Array Subset(array=w1956, new element=w1951, index (row)=23, index (col)=1) -> (w1937:string[][])
                n1035 = Replace Array Subset(array=w1937, new element=w1940, index (row)=0, index (col)=1) -> (w1936:string[][])
              }
              frame #1 {
                n1036 = Equal?(x=w2017, y=w2016) -> (x = y?=w2015:bool)
                n1037 = case shown="True" w2015 {
                  tunnel: w2017 -> [w2021 _]
                  tunnel: w2016 -> [w2020 _]
                  frame False {
                    n1038 = Move(source path=w2021, 9:TRUE, 10:w2020) -> ()  [unwired: 2 in, 3 out]
                  }
                  frame True {
                  }
                }
              }
              frame #2 {
                n1039 = local write "Data File"(w2023) -> ()
                n1040 = call-poly <vilib>:"Write To Spreadsheet File.vi"("2D data"=w2022, "file path (dialog if empty)"=w2023) -> ()  [unwired: 6 in, 1 out]
              }
              frame #3 {
                w2096 = 0
                # "Moves to next file and displays new image/data"
                n1041 = property on="Image Out" class="ImageControl"() -> (error out=w2058:errorcluster, "Image Center Position"=w2062:cluster{"X":u32, "Y":u32})  [unwired: 2 in, 1 out]
                n1042 = local read "Data File"() -> (w2101:path)
                n1043 = Strip Path(path=w2101) -> (stripped path=w2092:path, name=w2110:string)
                n1044 = Unbundle(w2062) -> ("X"=w2060:u32)  [unwired: 1 out]
                n1045 = local write "Data Folder"(w2092) -> ()
                n1046 = Bundle("X"=w2060, 0) -> (w2061:cluster{"X":u32, i32})  [unwired: 1 in]
                n1047 = property on="Image Out" class="ImageControl"(error in=w2058, "Image Center Position"=w2061) -> ()  [unwired: 1 in, 2 out]
                n1048 = List Folder(path=w2092) -> (filenames=w2106:string[])  [unwired: 3 in, 3 out]
                n1049 = Search 1D Array(1D array=w2106, element=w2110) -> (index of element=w2103:i32)  [unwired: 1 in]
                n1050 = Array Size(array=w2106) -> (size(s)=w2102:i32)
                n1051 = Decrement(x=w2102) -> (x-1=w2104:i32)
                n1052 = Equal?(x=w2103, y=w2104) -> (x = y?=w2105:bool)
                n1053 = local read "Folder Index"() -> (w2054:dbl)
                n1054 = case shown="False" w2105 {
                  tunnel: w2054 -> [w2233 _]
                  tunnel: [w2232 0] -> w2053
                  frame False {
                    n1055 = Increment(x=w2233) -> (x+1=w2232:dbl)
                  }
                  frame True {
                  }
                }
                n1056 = invoke on="Image Out" class="ImageControl" method="Clear ROI"() -> ()  [unwired: 3 in, 3 out]
                n1057 = local write "Folder Index"(w2053) -> ()
                n1058 = Path To String(path=w2092) -> (string=w2111:string)
                n1059 = Index Array(array=w2106, index=w2053) -> (element=w2107:string)
                n1060 = local write "Data Name:"(w2107) -> ()
                n1061 = Concatenate Strings(w2111, "\\", w2107) -> (w2109:string)
                n1062 = String To Path(string=w2109) -> (path=w2052:path)
                n1063 = local write "Data File"(w2052) -> ()
                n1064 = local read "NumPts 2"() -> (w2048:dbl)
                n1065 = local read "NumPts"() -> (w2037:dbl)
                n1066 = local read "NumPts"() -> (w2049:dbl)
                n1067 = call-poly <vilib>:"Read From Spreadsheet File.vi"("file path (dialog if empty)"=w2052) -> ("all rows"=w2098:string[][])  [unwired: 6 in, 4 out]
                n1068 = call "Mobility-Vt Calculator-File.vi"("NumPts"=w2049, "Path"=w2052) -> ("XY Graph-Sat"=w2050:cluster{dbl[], dbl[]}[], "XY Graph-Lin"=w2032:cluster{dbl[], dbl[]}[], "Output"=w2051:T8, "Index-Sat"=w2027:dbl, "Index-Lin"=w2036:dbl)  [unwired: 4 in, 1 out]
                n1069 = Decimate 1D Array(w2032) -> (w2044:cluster{dbl[], dbl[]}[])  [unwired: 1 out]
                n1070 = Array To Cluster(array=w2044) -> (cluster=w2042:T9)
                n1071 = Unbundle(w2042) -> ("[0]"=w2043:cluster{dbl[], dbl[]})  [unwired: 8 out]
                n1072 = local write "XY Graph-Lin"(w2032) -> ()
                n1073 = Unbundle(w2043) -> (w2041:dbl[], w2040:dbl[])
                n1074 = Array Subset(array=w2040, index=w2036, length=w2037) -> (w2038:dbl[])
                n1075 = Array Subset(array=w2041, index=w2036, length=w2037) -> (w2039:dbl[])
                n1076 = call "STS Calculator-File.vi"("NumPts"=w2048, "Path"=w2052) -> ("STS Index-Sat"=w2047:dbl, "XY Graph-Sat"=w2046:cluster{dbl[], dbl[]}[], "Ouput"=w2045:cluster{"STS-Sat":dbl, "STS-Lin":dbl})  [unwired: 5 in, 2 out]
                n1077 = local read "New: Dielectric"() -> (w2031:dbl)
                n1078 = local read "New: Temp"() -> (w2030:dbl)
                n1079 = local write "Lin Id-Used"(w2038) -> ()
                n1080 = local write "Lin-Vg Array-Used"(w2039) -> ()
                n1081 = local write "MobVi Index"(w2027) -> ()
                n1082 = local write "Slide"(w2027) -> ()
                n1083 = local write "XY Graph"(w2050) -> ()
                n1084 = local write "Index 2"(w2047) -> ()
                n1085 = local write "XY Graph 2"(w2046) -> ()
                n1086 = Unbundle By Name(w2051) -> ("Mobility-Sat"=w2035:dbl, "Vt-Sat"=w2026:dbl, "Mobility-Lin"=w2034:dbl, "Mobility-Lin"=w2033:dbl)
                n1087 = Array Size(array=w2098) -> (size(s)=w2097:i32[])
                n1088 = Unbundle By Name(w2045) -> ("STS-Sat"=w2029:dbl)
                n1089 = call "Trap Density_STS.vi"("Temp (T) [K]"=w2030, "S.T.S. (S)"=w2029, "Dielectric"=w2031) -> ("Trap Density (N)"=w2028:dbl)  [unwired: 8 in]
                n1090 = local write "Calc: Mobility-Sat"(w2035) -> ()
                n1091 = local write "Calc: Mobility-Lin"(w2033) -> ()
                n1092 = local write "New: Trap Density-STS"(w2028) -> ()
                n1093 = local read "Image Folder"() -> (w2086:path)
                n1094 = local write "Calc: VT-Sat"(w2026) -> ()
                n1095 = local write "Calc: VT-Lin"(w2034) -> ()
                n1096 = local read "New: Dielectric"() -> (w2024:dbl)
                n1097 = Decimate 1D Array(w2050) -> (w2081:cluster{dbl[], dbl[]}[])  [unwired: 1 out]
                n1098 = Index Array(array=w2097, index=w2096) -> (element=w2077:i32)
                n1099 = Decimate 1D Array(w2046) -> (w2071:cluster{dbl[], dbl[]}[])  [unwired: 1 out]
                n1100 = Array Subset(array=w2098, index (row)=w2096, index (col)=w2096, length (col)=3) -> (w2099:string[][])  [unwired: 1 in]
                n1101 = local write "Calc: STS"(w2029) -> ()
                n1102 = List Folder(path=w2086) -> (filenames=w2091:string[])  [unwired: 3 in, 3 out]
                n1103 = local write "New: Mobility-Sat"(w2035) -> ()
                n1104 = Array To Cluster(array=w2081) -> (cluster=w2083:T9)
                n1105 = Array To Cluster(array=w2071) -> (cluster=w2069:T9)
                n1106 = Reshape Array(w2099, w2077) -> (w2084:string[])
                n1107 = local write "New: Mobility-Lin"(w2034) -> ()
                n1108 = Subtract(x=w2077, y=20) -> (x-y=w2076:i32)
                n1109 = local write "New: VT-Sat"(w2026) -> ()
                n1110 = local write "New: VT-Lin"(w2033) -> ()
                n1111 = local write "New: STS"(w2029) -> ()
                n1112 = property on="Slide" class="Slide (strict)"("Scale.Maximum"=w2076) -> ()  [unwired: 2 in, 2 out]
                n1113 = call "Trap Density_VT.vi"("VT"=w2026, "Dielectric"=w2024) -> ("Trap Density-VT"=w2025:dbl)
                n1114 = Unbundle(w2083) -> ("[0]"=w2082:cluster{dbl[], dbl[]})  [unwired: 8 out]
                n1115 = Unbundle(w2069) -> ("[0]"=w2070:cluster{dbl[], dbl[]})  [unwired: 8 out]
                n1116 = Search 1D Array(1D array=w2084, element="Index:") -> (index of element=w2093:i32)  [unwired: 1 in]
                n1117 = local write "New: Trap Density-VT"(w2025) -> ()
                n1118 = Increment(x=w2093) -> (x+1=w2094:i32)
                n1119 = Unbundle(w2082) -> (w2073:dbl[], w2072:dbl[])
                n1120 = Unbundle(w2070) -> (w2068:dbl[], w2067:dbl[])
                n1121 = Array Subset(array=w2073, index=w2027, length=w2049) -> (w2080:dbl[])
                n1122 = Array Subset(array=w2072, index=w2027, length=w2049) -> (w2079:dbl[])
                n1123 = Array Subset(array=w2068, index=w2047, length=w2048) -> (w2075:dbl[])
                n1124 = Array Subset(array=w2067, index=w2047, length=w2048) -> (w2074:dbl[])
                n1125 = Index Array(array=w2084, index=w2094) -> (element=w2089:string)
                n1126 = local write "Vg Array-Log-Used"(w2074) -> ()
                n1127 = local write "Sat Id-Log-Used"(w2075) -> ()
                n1128 = local write "Sat Id-Used"(w2079) -> ()
                n1129 = local write "Index"(w2089) -> ()
                n1130 = local write "Sat Vg Array-Used"(w2080) -> ()
                n1131 = while {
                  tunnel: w2091 -> [w2119]
                  tunnel: w2089 -> [w2117]
                  tunnel: [w2116] -> _
                  tunnel: [w2116] -> w2090
                  tunnel: w2077 -> [w2115]
                  i -> [w2116]
                  stop <- w2112 stop-if-true
                  n1132 = Index Array(array=w2119, index=w2116) -> (element=w2120:string)
                  n1133 = xnode "Match Regular Expression"("input string"=w2120, "regular expression"=w2117) -> ("whole match"=w2118:string)  [unwired: 4 in, 4 out]
                  n1134 = Equal?(x=w2118, y=w2117) -> (x = y?=w2114:bool)
                  n1135 = Equal?(x=w2115, y=w2116) -> (x = y?=w2113:bool)
                  n1136 = Or(x=w2114, y=w2113) -> (x .or. y?=w2112:bool)
                }
                n1137 = Path To String(path=w2086) -> (string=w2088:string)
                n1138 = Index Array(array=w2091, index=w2090) -> (element=w2065:string)
                n1139 = local write "Image Name"(w2065) -> ()
                n1140 = Empty String/Path?(string/path=w2065) -> (empty?=w2066:bool)
                n1141 = Concatenate Strings(w2088, "\\", w2065) -> (w2087:string)
                n1142 = String To Path(string=w2087) -> (path=w2064:path)
                n1143 = local read "No Image"() -> (w2063:path)
                n1144 = Select(t=w2063, s=w2066, f=w2064) -> (s? t:f=w2057:path)
                n1145 = local write "Image File"(w2057) -> ()
                n1146 = local read "Image Out"() -> (w2055:T2)
                n1147 = call "IMAQ ReadFile"("File Path"=w2057, "Image"=w2055) -> ("Image Out"=w2056:T2)  [unwired: 5 in, 4 out]
                n1148 = local write "Image Out"(w2056) -> ()
                n1149 = local write "Image Out 2"(w2056) -> ()
              }
              frame #4 {
                # "Output ROI data"
                n1150 = local read "Image Folder"() -> (w2235:path)
                n1151 = Build Path(base path=w2235, name or relative path="ROI") -> (appended path=w2237:path)
                n1152 = local read "Index"() -> (w2236:string)
                n1153 = Build Path(base path=w2237, name or relative path=w2236) -> (appended path=w2242:path)
                n1154 = invoke on="Image Out" class="ImageControl" method="Clear ROI"() -> (error out=w2241:errorcluster)  [unwired: 3 in, 2 out]
                n1155 = call <vilib>:"Check if File or Folder Exists.vi"("error in (no error)"=w2241, "path"=w2242) -> ("file or folder exists?"=w2239:bool, "dup path"=w2240:path)  [unwired: 7 in, 1 out]
                n1156 = case shown="True" w2239 {
                  tunnel: w2240 -> [_ w2243]
                  frame False {
                  }
                  frame True {
                    n1157 = Read from Text File(file (use dialog)=w2243) -> (text=w2247:string)  [unwired: 3 in, 3 out]
                    n1158 = property on="Image Out" class="ImageControl"() -> ("ROI"=w2244:T10)  [unwired: 2 in, 2 out]
                    n1159 = Unflatten From String(type=w2244, binary string=w2247) -> (value=w2245:T10, error out=w2246:errorcluster)  [unwired: 3 in, 1 out]
                    n1160 = property on="Image Out" class="ImageControl"(error in=w2246, "ROI"=w2245) -> ()  [unwired: 1 in, 2 out]
                  }
                }
              }
            }
            n1161 = flat-sequence {
              tunnel: [w1893] -> w1880
              tunnel: w1880 -> [w1907]
              frame #0 {
                # "Makes Empty File for Transformer Data"
                n1162 = local read "Data Folder"() -> (w1882:path)
                n1163 = Build Path(base path=w1882, name or relative path="Stats") -> (appended path=w1884:path)
                n1164 = call <vilib>:"Check if File or Folder Exists.vi"("path"=w1884) -> ("file or folder exists?"=w1885:bool, "dup path"=w1886:path)  [unwired: 8 in, 1 out]
                n1165 = case shown="False" w1885 {
                  tunnel: [w1890 w1892] -> w1887
                  tunnel: w1886 -> [w1891 w1892]
                  frame False {
                    n1166 = Create Folder(path (use dialog)=w1891) -> (created path=w1890:path)  [unwired: 2 in, 2 out]
                  }
                  frame True {
                  }
                }
                n1167 = Build Path(base path=w1887, name or relative path="Tranformer Data.txt") -> (appended path=w1889:path)
                n1168 = call-poly <vilib>:"Write To Spreadsheet File.vi"("append to file? (new file:F)"=TRUE, "file path (dialog if empty)"=w1889) -> ()  [unwired: 6 in, 1 out]
              }
              frame #1 {
                # "Adds Headers if they don't exist"
                n1169 = Concatenate Strings("Stats\\", "Tranformer Data.txt") -> (w1900:string)
                n1170 = local read "Data Folder"() -> (w1899:path)
                n1171 = Build Path(base path=w1899, name or relative path=w1900) -> (appended path=w1893:path)
                n1172 = call-poly <vilib>:"Read From Spreadsheet File.vi"("file path (dialog if empty)"=w1893) -> ("first row"=w1898:string[])  [unwired: 6 in, 4 out]
                n1173 = Search 1D Array(1D array=w1898, element="DeviceID") -> (index of element=w1896:i32)  [unwired: 1 in]
                n1174 = Equal?(x=w1896, y=0) -> (x = y?=w1894:bool)
                n1175 = case shown="False" w1894 {
                  tunnel: w1893 -> [w1904 _]
                  frame False {
                    n1176 = local read "Transformer \nHeaders"() -> (w1903:string[])
                    n1177 = call-poly <vilib>:"Write To Spreadsheet File.vi"("1D data"=w1903, "file path (dialog if empty)"=w1904) -> ()  [unwired: 6 in, 1 out]
                  }
                  frame True {
                  }
                }
              }
              frame #2 {
                # "Adds current device if it doesn't exist"
                n1178 = local read "Current \nRecord"() -> (w1910:string[])
                n1179 = Index Array(array=w1910, index=0) -> (element=w1909:string)
                n1180 = Concatenate Strings("Stats\\", "Tranformer Data.txt") -> (w1913:string)
                n1181 = local read "Data Folder"() -> (w1912:path)
                n1182 = local write "Current Device ID"(w1909) -> ()
                n1183 = local read "Current Device ID"() -> (w1919:string)
                n1184 = Build Path(base path=w1912, name or relative path=w1913) -> (appended path=w1911:path)
                n1185 = call-poly <vilib>:"Read From Spreadsheet File.vi"("file path (dialog if empty)"=w1911) -> ("all rows"=w1906:string[][])  [unwired: 6 in, 4 out]
                n1186 = Index Array(array=w1906, index (col)=0) -> (element=w1917:string[])  [unwired: 1 in]
                n1187 = Search 1D Array(1D array=w1917, element=w1919) -> (index of element=w1905:i32)  [unwired: 1 in]
                n1188 = Equal?(x=w1905, y=-1) -> (x = y?=w1908:bool)
                n1189 = case shown="False" w1908 {
                  tunnel: w1907 -> [w1921 w1934]
                  tunnel: w1905 -> [w1926 _]
                  tunnel: w1906 -> [w1927 _]
                  frame False {
                    n1190 = local read "Current \nRecord"() -> (w1925:string[])
                    n1191 = Replace Array Subset(array=w1927, new element=w1925, index (row)=w1926) -> (w1922:string[][])  [unwired: 1 in]
                    n1192 = flat-sequence {
                      tunnel: [w1928] -> _
                      tunnel: [w1929] -> _
                      tunnel: [w1929] -> w1924
                      tunnel: [w1928] -> w1923
                      tunnel: w1922 -> [w1929]
                      tunnel: w1921 -> [w1928]
                      tunnel: w1924 -> [w1931]
                      tunnel: w1923 -> [w1930]
                      frame #0 {
                        n1193 = Delete(path (use dialog)=w1928) -> ()  [unwired: 4 in, 3 out]
                      }
                      frame #1 {
                        n1194 = call-poly <vilib>:"Write To Spreadsheet File.vi"("append to file? (new file:F)"=TRUE, "2D data"=w1931, "file path (dialog if empty)"=w1930) -> ()  [unwired: 5 in, 1 out]
                      }
                    }
                  }
                  frame True {
                    n1195 = local read "Current \nRecord"() -> (w1933:string[])
                    n1196 = call-poly <vilib>:"Write To Spreadsheet File.vi"("append to file? (new file:F)"=TRUE, "1D data"=w1933, "file path (dialog if empty)"=w1934) -> ()  [unwired: 5 in, 1 out]
                  }
                }
              }
            }
          }
          event "Export": Mouse Down {
            n1197 = event-data() -> ()  [unwired: 1 in, 7 out]
            n1198 = call "OA_ConnectToOrigin.vi"() -> ("error out"=w2271:errorcluster, "Origin.IOApplication"=w2272:refnum<k7>)  [unwired: 8 in]
            n1199 = local read "Data Folder"() -> (w2249:path)
            n1200 = local read "Project"() -> (w2270:path)
            n1201 = call "OA_Load.vi"("error in (no error)"=w2271, "Path"=w2270, "Origin.IOApplication"=w2272) -> ("error out"=w2264:errorcluster, "Origin.IOApplication"=w2265:refnum<k7>)  [unwired: 1 out]
            n1202 = call "OAExecute.vi"("script"="document -m 3;", "Error IO"=w2264, "Origin.IOApplication"=w2265) -> ("Error IO Out"=w2262:errorcluster, "Origin.IOApplication"=w2263:refnum<k7>)  [unwired: 1 in, 1 out]
            n1203 = Build Path(base path=w2249, name or relative path="Stats") -> (appended path=w2252:path)
            n1204 = flat-sequence {
              tunnel: w2249 -> [w2292]
              tunnel: w2248 -> [w2291]
              tunnel: [w2281] -> w2274
              tunnel: [w2282] -> w2273
              tunnel: w2263 -> [w2286]
              tunnel: w2262 -> [w2285]
              tunnel: w2249 -> [w2308]
              tunnel: w2248 -> [w2307]
              tunnel: w2274 -> [w2303]
              tunnel: w2273 -> [w2304]
              tunnel: [w2298] -> w2269
              tunnel: [w2297] -> w2268
              tunnel: w2249 -> [w2319]
              tunnel: w2248 -> [w2318]
              tunnel: w2269 -> [w2314]
              tunnel: w2268 -> [w2313]
              tunnel: [w2312] -> w2267
              tunnel: [w2311] -> w2266
              tunnel: w2249 -> [w2334]
              tunnel: w2248 -> [w2333]
              tunnel: w2267 -> [w2328]
              tunnel: w2266 -> [w2327]
              tunnel: [w2325] -> w2251
              tunnel: [w2324] -> w2250
              tunnel: [w2335] -> w2259
              tunnel: [w2336] -> w2260
              tunnel: w2251 -> [w2338]
              tunnel: w2250 -> [w2337]
              tunnel: w2249 -> [w2340]
              tunnel: w2248 -> [w2339]
              frame #0 {
                n1205 = call "Param_Analysis.vi"("error in (no error)"=w2285, "Data Folder"=w2292, "Parameter String"="Mobility (cm^2/Vs):", "Parameter Name"="Mobility", "Stats Folder"=w2291) -> ("error out"=w2288:errorcluster, "Array 4"=w2278:string[], "Array 3"=w2287:string[][])  [unwired: 3 in, 1 out]
                n1206 = call "Origin_Export.vi"("String 3"="[MobHistTab]Sheet1", "error in (no error)"=w2288, "Array"=w2287, "String 2"="[MOBvsLTable]Mobilities", "String"="pe_cd \"Mobility Chart\";", "Origin.IOApplication"=w2286, "Array 2"=w2278) -> ("reference out"=w2284:refnum<k7>, "error out"=w2283:errorcluster)  [unwired: 2 in, 1 out]
                n1207 = call "OAExecute.vi"("script"="window -a MOBvsLTable;\nwindow -s TV;", "Error IO"=w2283, "Origin.IOApplication"=w2284) -> ("Error IO Out"=w2281:errorcluster, "Origin.IOApplication"=w2282:refnum<k7>)  [unwired: 1 in, 1 out]
              }
              frame #1 {
                n1208 = call "Param_Analysis.vi"("error in (no error)"=w2303, "Data Folder"=w2308, "Parameter String"="On/Off Current:", "Parameter Name"="On_Off_Current", "Stats Folder"=w2307) -> ("error out"=w2302:errorcluster, "Array 4"=w2296:string[], "Array 3"=w2299:string[][])  [unwired: 3 in, 1 out]
                n1209 = call "Origin_Export.vi"("String 3"="[OnOffHistTab]Sheet1", "error in (no error)"=w2302, "Array"=w2299, "String 2"="[OnOffTable]On/Off Ratios", "String"="pe_cd \"OnOff vs L\";", "Origin.IOApplication"=w2304, "Array 2"=w2296) -> ("reference out"=w2298:refnum<k7>, "error out"=w2297:errorcluster)  [unwired: 2 in, 1 out]
              }
              frame #2 {
                n1210 = call "Param_Analysis.vi"("Data Folder"=w2319, "Parameter String"="S.T.S. (V/decade):", "Parameter Name"="STS", "Stats Folder"=w2318) -> ("Array 4"=w2310:string[], "Array 3"=w2315:string[][])  [unwired: 4 in, 2 out]
                n1211 = call "Origin_Export.vi"("String 3"="[SHistTab]Sheet1", "error in (no error)"=w2313, "Array"=w2315, "String 2"="[STable]Threshold Swing", "String"="pe_cd \"Threshold Swing vs L\";", "Origin.IOApplication"=w2314, "Array 2"=w2310) -> ("reference out"=w2311:refnum<k7>, "error out"=w2312:errorcluster)  [unwired: 2 in, 1 out]
              }
              frame #3 {
                n1212 = call "Param_Analysis.vi"("Data Folder"=w2334, "Parameter String"="Threshold V (V):", "Parameter Name"="Threshold_V", "Stats Folder"=w2333) -> ("Array 4"=w2323:string[], "Array 3"=w2326:string[][])  [unwired: 4 in, 2 out]
                n1213 = call "Origin_Export.vi"("String 3"="[VtHistTab]Sheet1", "error in (no error)"=w2328, "Array"=w2326, "String 2"="[VtTable]Threshold Voltages", "String"="pe_cd \"Threshold Voltage vs L\";", "Origin.IOApplication"=w2327, "Array 2"=w2323) -> ("reference out"=w2325:refnum<k7>, "error out"=w2324:errorcluster)  [unwired: 2 in, 1 out]
              }
              frame #4 {
                n1214 = call "Param_Analysis.vi"("Data Folder"=w2340, "Parameter String"="Off I-Sat (A):", "Parameter Name"="OffI_Sat", "Stats Folder"=w2339) -> ("Array 4"=w2346:string[], "Array 3"=w2345:string[][])  [unwired: 4 in, 2 out]
                n1215 = call "Origin_Export.vi"("String 3"=" ", "error in (no error)"=w2337, "Array"=w2345, "String 2"=" ", "String"=" ", "Origin.IOApplication"=w2338, "Array 2"=w2346) -> ("reference out"=w2336:refnum<k7>, "error out"=w2335:errorcluster)  [unwired: 2 in, 1 out]
              }
            }
            n1216 = call <vilib>:"Check if File or Folder Exists.vi"("path"=w2252) -> ("file or folder exists?"=w2276:bool, "dup path"=w2275:path)  [unwired: 8 in, 1 out]
            n1217 = case shown="False" w2276 {
              tunnel: w2275 -> [w2349 w2350]
              tunnel: [w2348 w2350] -> w2248
              frame False {
                n1218 = Create Folder(path (use dialog)=w2349) -> (created path=w2348:path)  [unwired: 2 in, 2 out]
              }
              frame True {
              }
            }
            n1219 = call "File Dialog"("start path"=w2252) -> ("selected path"=w2255:path)  [unwired: 11 in, 3 out]
            n1220 = Path To String(path=w2255) -> (string=w2254:string)
            n1221 = call "OAExecute.vi"("script"="pe_cd /;\npe_cd \"Mobility Chart\"; ", "Error IO"=w2259, "Origin.IOApplication"=w2260) -> ("Error IO Out"=w2256:errorcluster, "Origin.IOApplication"=w2257:refnum<k7>)  [unwired: 1 in, 1 out]
            n1222 = call "OASaveProject.vi"("path"=w2254, "Error IO"=w2256, "Origin.IOApplication"=w2257) -> ()  [unwired: 3 out]
          }
          event "Blank Button": Mouse Down {
            n1223 = event-data() -> ()  [unwired: 1 in, 7 out]
            n1224 = local read "Data File"() -> (w2358:path)
            n1225 = Strip Path(path=w2358) -> (stripped path=w2354:path, name=w2356:string)
            n1226 = Path To String(path=w2354) -> (string=w2353:string)
            n1227 = Concatenate Strings(w2353, "\\", "X_", w2356) -> (w2352:string)
            n1228 = String To Path(string=w2352) -> (path=w2351:path)
            n1229 = Move(source path=w2358, 10:w2351) -> ()  [unwired: 3 in, 3 out]
            n1230 = local write "Data File"(w2351) -> ()
          }
          event "Cancel Button": Mouse Down {
            (unwired) 6
            n1231 = event-data() -> ()  [unwired: 1 in, 7 out]
            n1232 = call "Simulate_Keyboard.vi"("Action"=2, "Virtual Key"=162) -> ()  [unwired: 7 in, 1 out]
          }
        }
        n1233 = Reciprocal(x=w516) -> (1/x=w515:sgl)
        n1234 = Multiply(x=w515, y=10) -> (x*y=w517:sgl)
        n1235 = case shown="\"EQUALS\"" w556 {
          tunnel: w530 -> [w607 w613 w617 w619 w623 w625 w627 w629 w631 w633 w635 w637 w639 w641 w643 w645 w647 w649 w651 w653 w655 w657 w659 w661 w663 w665 w667 w669 w671 w673 w675 w677 w679 w681 w683 w685 w687 w689 w691 w693 w695 w697 w699 w701 w703 w705 w707 w709 w711 w713 w715 w717 w719 w721 w723 w725 w727 w729 w731 w733 w735 w737 w739 w741 w743 w745 w747 w749 w751 w753 w755 w757 w759 w761 w763 w765 w767 w769 w771 w773 w775 w777 w779 w781 w783 w785 w787 w789 w791 w793 w795 w797 w799 w801 w803 w805 w807 w809 w811 w813 w815 w817 w819 w821 w823]
          tunnel: [w607 w612 w616 w619 w623 w625 w627 w629 w631 w633 w635 w637 w639 w641 w643 w645 w647 w649 w651 w653 w655 w657 w659 w661 w663 w665 w667 w669 w671 w673 w675 w677 w679 w681 w683 w685 w687 w689 w691 w693 w695 w697 w699 w701 w703 w705 w707 w709 w711 w713 w715 w717 w719 w721 w723 w725 w727 w729 w731 w733 w735 w737 w739 w741 w743 w745 w747 w749 w751 w753 w755 w757 w759 w761 w763 w765 w767 w769 w771 w773 w775 w777 w779 w781 w783 w785 w787 w789 w791 w793 w795 w797 w799 w801 w803 w805 w807 w809 w811 w813 w815 w817 w819 w821 w823] -> w555
          tunnel: w531 -> [w609 w611 w615 w621 w622 w624 w626 w628 w630 w632 w634 w636 w638 w640 w642 w644 w646 w648 w650 w652 w654 w656 w658 w660 w662 w664 w666 w668 w670 w672 w674 w676 w678 w680 w682 w684 w686 w688 w690 w692 w694 w696 w698 w700 w702 w704 w706 w708 w710 w712 w714 w716 w718 w720 w722 w724 w726 w728 w730 w732 w734 w736 w738 w740 w742 w744 w746 w748 w750 w752 w754 w756 w758 w760 w762 w764 w766 w768 w770 w772 w774 w776 w778 w780 w782 w784 w786 w788 w790 w792 w794 w796 w798 w800 w802 w804 w806 w808 w810 w812 w814 w816 w818 w820 w822]
          tunnel: [w608 w611 w615 w620 w622 w624 w626 w628 w630 w632 w634 w636 w638 w640 w642 w644 w646 w648 w650 w652 w654 w656 w658 w660 w662 w664 w666 w668 w670 w672 w674 w676 w678 w680 w682 w684 w686 w688 w690 w692 w694 w696 w698 w700 w702 w704 w706 w708 w710 w712 w714 w716 w718 w720 w722 w724 w726 w728 w730 w732 w734 w736 w738 w740 w742 w744 w746 w748 w750 w752 w754 w756 w758 w760 w762 w764 w766 w768 w770 w772 w774 w776 w778 w780 w782 w784 w786 w788 w790 w792 w794 w796 w798 w800 w802 w804 w806 w808 w810 w812 w814 w816 w818 w820 w822] -> w554
          tunnel: w517 -> [w606 w610 w614 w618 _ _ _ _ _ _ _ _ _ _ _ _ _ _ _ _ _ _ _ _ _ _ _ _ _ _ _ _ _ _ _ _ _ _ _ _ _ _ _ _ _ _ _ _ _ _ _ _ _ _ _ _ _ _ _ _ _ _ _ _ _ _ _ _ _ _ _ _ _ _ _ _ _ _ _ _ _ _ _ _ _ _ _ _ _ _ _ _ _ _ _ _ _ _ _ _ _ _ _ _ _]
          frame "DOWN" {
            n1236 = Add(x=w609, y=w606) -> (x+y=w608:sgl)
          }
          frame "LEFT" {
            n1237 = Subtract(x=w613, y=w610) -> (x-y=w612:sgl)
          }
          frame "RIGHT" {
            n1238 = Add(x=w617, y=w614) -> (x+y=w616:sgl)
          }
          frame "UP" {
            n1239 = Subtract(x=w621, y=w618) -> (x-y=w620:sgl)
          }
          frame "ENTER (num pad)" {
          }
          frame "' (quote)" {
          }
          frame "END" {
          }
          frame "EQUALS" {
          }
          frame "ESCAPE" {
          }
          frame "GRAVE (`)" {
          }
          frame "HOME" {
          }
          frame "INSERT" {
          }
          frame "LBRACKET" {
          }
          frame "LCONTROL" {
          }
          frame "L ALT" {
          }
          frame "LSHIFT" {
          }
          frame "LWIN" {
          }
          frame "MINUS" {
          }
          frame "MULTIPLY" {
          }
          frame "NEXT" {
          }
          frame "NUMLOCK" {
          }
          frame "NUMPAD_0" {
          }
          frame "NUMPAD_1" {
          }
          frame "NUMPAD_2" {
          }
          frame "NUMPAD_3" {
          }
          frame "NUMPAD_4" {
          }
          frame "NUMPAD_5" {
          }
          frame "NUMPAD_6" {
          }
          frame "NUMPAD_7" {
          }
          frame "NUMPAD_8" {
          }
          frame "NUMPAD_9" {
          }
          frame "PAUSE" {
          }
          frame "PERIOD" {
          }
          frame "PRIOR (PG UP)" {
          }
          frame "RBRACKET" {
          }
          frame "RCONTROL" {
          }
          frame "RETURN" {
          }
          frame "R ALT" {
          }
          frame "RSHIFT" {
          }
          frame "RWIN" {
          }
          frame "SCROLL" {
          }
          frame "SEMICOLON" {
          }
          frame "SLASH" {
          }
          frame "SPACE" {
          }
          frame "SUBTRACT" {
          }
          frame "TAB" {
          }
          frame "DIVIDE" {
          }
          frame "DELETE" {
          }
          frame "DECIMAL" {
          }
          frame "COMMA" {
          }
          frame "CAPITAL" {
          }
          frame "BACKSLASH" {
          }
          frame "BACK" {
          }
          frame "ADD" {
          }
          frame "F15" {
          }
          frame "F14" {
          }
          frame "F13" {
          }
          frame "F12" {
          }
          frame "F11" {
          }
          frame "F10" {
          }
          frame "F9" {
          }
          frame "F8" {
          }
          frame "F7" {
          }
          frame "F6" {
          }
          frame "F5" {
          }
          frame "F4" {
          }
          frame "F3" {
          }
          frame "F2" {
          }
          frame "F1" {
          }
          frame "Z" {
          }
          frame "Y" {
          }
          frame "X" {
          }
          frame "W" {
          }
          frame "V" {
          }
          frame "U" {
          }
          frame "T" {
          }
          frame "S" {
          }
          frame "R" {
          }
          frame "Q" {
          }
          frame "P" {
          }
          frame "O" {
          }
          frame "N" {
          }
          frame "M" {
          }
          frame "L" {
          }
          frame "K" {
          }
          frame "J" {
          }
          frame "I" {
          }
          frame "H" {
          }
          frame "G" {
          }
          frame "F" {
          }
          frame "E" {
          }
          frame "D" {
          }
          frame "C" {
          }
          frame "B" {
          }
          frame "A" {
          }
          frame "9" {
          }
          frame "8" {
          }
          frame "7" {
          }
          frame "6" {
          }
          frame "5" {
          }
          frame "4" {
          }
          frame "3" {
          }
          frame "2" {
          }
          frame "1" {
          }
          frame "0" {
          }
        }
        n1240 = Bundle(w533, w532, w547, w546, 0.0) -> (w545:cluster{dbl, dbl, dbl, dbl, dbl})  [unwired: 1 in]
        n1241 = Bundle("X"=w555, "Y"=w554) -> (w549:cluster{"X":sgl, "Y":sgl})  [unwired: 1 in]
        n1242 = Divide(x=20, y=w516) -> (x/y=w519:sgl)
        n1243 = property on="Image Out" class="ImageControl"("Image Center Position"=w549) -> ()  [unwired: 2 in, 2 out]
        n1244 = call "IMAQ Convert Rectangle to ROI (Polygon)"("Rectangle"=w545) -> ("ROI Descriptor"=w543:T3)  [unwired: 7 in, 2 out]
        n1245 = Bundle("Application Font", w519, w523, w523, w523, w523, w523, TRUE, w521) -> (w525:T16)  [unwired: 1 in]
        n1246 = property on="Image Out 2" class="ImageControl"("ROI"=w543) -> ()  [unwired: 2 in, 2 out]
        n1247 = Bundle(w521, w525, w521, w521) -> (w524:T17)  [unwired: 1 in]
        n1248 = property on="Image Out" class="ImageControl"() -> ("ROI"=w508:T10)  [unwired: 2 in, 2 out]
        n1249 = Unbundle By Name(w508) -> ("Contours"=w572:T14)
        n1250 = local read "Image Out"() -> (w527:T2)
        n1251 = call "IMAQ Clear Overlay"("Image"=w527) -> ("Image Out"=w526:T2)  [unwired: 9 in, 1 out]
        n1252 = Initialize Array(0) -> (w570:i32[])  [unwired: 1 in]
        n1253 = local read "Magnification"() -> (w561:u16)
        n1254 = Array Size(array=w572) -> (size(s)=w571:i32)
        n1255 = Build Array(0.505025, 0.252522, 0.127742, 0.050345, 0.031129) -> (w562:dbl[])
        n1256 = Array Subset(array=w562, index=w561, length=1) -> (w559:dbl[])
        n1257 = property on="Image Out" class="ImageControl"() -> ("ZoomInteger"=w551:cluster{"X":i32, "Y":i32})  [unwired: 2 in, 2 out]
        n1258 = To Double Precision Float(number=w559) -> (double precision float=w558:dbl[])
        n1259 = for {
          N: w571 -> [_]
          shift-right: [w846] -> _
          shift-left: w572 -> [w846]
          shift-right: [w844] -> w557
          shift-left: w570 -> [w843]
          tunnel: w558 -> [w842]
          shift-right: [w839] -> _
          shift-left: w526 -> [w841]
          tunnel: w524 -> [w834]
          i -> [w838]
          n1260 = Index Array(array=w846, index=w838) -> (element=w855:T18)
          n1261 = Unbundle(w855) -> ("Points"=w854:i32[])  [unwired: 2 out]
          n1262 = Array To Cluster(array=w854) -> (cluster=w853:T19)
          n1263 = Unbundle(w853) -> ("Points[0]"=w833:i32, "Points[1]"=w830:i32, "Points[2]"=w845:i32, "Points[3]"=w851:i32)  [unwired: 5 out]
          n1264 = Add(x=w833, y=10) -> (x+y=w831:i32)
          n1265 = Subtract(x=w830, y=w851) -> (x-y=w850:i32)
          n1266 = Subtract(x=w833, y=w845) -> (x-y=w852:i32)
          n1267 = Square(x=w850) -> (x^2=w848:i32)
          n1268 = Square(x=w852) -> (x^2=w849:i32)
          n1269 = Add(x=w849, y=w848) -> (x+y=w847:i32)
          n1270 = Square Root(x=w847) -> (sqrt(x)=w824:dbl)
          n1271 = Multiply(x=w824, y=0.5) -> (x*y=w827:dbl)
          n1272 = Add(x=w827, y=w830) -> (x+y=w829:dbl)
          n1273 = Bundle(w831, w829) -> (w840:cluster{i32, dbl})  [unwired: 1 in]
          n1274 = Multiply(x=w824, y=w842) -> (x*y=w837:dbl[])
          n1275 = Index Array(array=w837) -> (element=w836:dbl)  [unwired: 1 in]
          n1276 = Number To Fractional String(number=w836) -> (F-format string=w835:string)  [unwired: 3 in]
          n1277 = call "IMAQ Overlay Text"("BG Color (Transparent)"=u32 0, "Text Color (black)"=u32 16448250, "Font, Size & Style"=w834, "String"=w835, "Origin"=w840, "Image"=w841) -> ("Image Out"=w839:T2)  [unwired: 4 in, 1 out]
          n1278 = Build Array (concatenate)(w843, w837) -> (w844:dbl[])
          n1279 = local write "Numeric 3"(w824) -> ()
        }
        n1280 = local write "ROI Descriptor"(w508) -> ()
        n1281 = Unbundle(w551) -> ("X"=w550:i32)  [unwired: 1 out]
        n1282 = Add Array Elements(numeric array=w557) -> (sum=w568:dbl)
        n1283 = local write "Distances"(w557) -> ()
        n1284 = local write "Total Width"(w568) -> ()
        n1285 = local write "Zoom"(w550) -> ()
        n1286 = local read "Total Width"() -> (w511:dbl)
        n1287 = local read "Rec: Width"() -> (w509:dbl)
        n1288 = local read "Manual-Width"() -> (w507:bool)
        n1289 = Not(x=w507) -> (.not. x?=w505:bool)
        n1290 = Equal To 0?(x=w511) -> (x = 0?=w506:bool)
        n1291 = Or(x=w506, y=w507) -> (x .or. y?=w510:bool)
        n1292 = And(x=w506, y=w505) -> (x .and. y?=w504:bool)
        n1293 = case shown="True" w504 {
          tunnel: w509 -> [_ w584]
          frame False {
          }
          frame True {
            n1294 = local write "New: Width"(w584) -> ()
          }
        }
        n1295 = case shown="False" w510 {
          tunnel: w511 -> [w585 _]
          frame False {
            n1296 = local write "New: Width"(w585) -> ()
          }
          frame True {
          }
        }
        n1297 = local read "Manuel-Dielectric"() -> (w433:bool)
        n1298 = local read "Rec: Dielectric (d)"() -> (w432:dbl)
        n1299 = local read "Manuel-Length"() -> (w434:bool)
        n1300 = local read "Rec: Length"() -> (w435:dbl)
        n1301 = case shown="False" w434 {
          tunnel: w435 -> [w575 _]
          frame False {
            n1302 = local write "New: Length"(w575) -> ()
          }
          frame True {
          }
        }
        n1303 = case shown="False" w433 {
          tunnel: w432 -> [w574 _]
          frame False {
            n1304 = local write "New: Dielectric"(w574) -> ()
          }
          frame True {
          }
        }
      }
    }
  }
  n1305 = Build Array("DeviceID", "Fabricator", "Deposition", "Date", "Sample", "Row", "Column", "L (um)", "W (um)", "Material", "Treatment", "TC (mM)", "Solvent", "C (%)", "ST (C)", "Drops", "Wait (s)", "RT (F)", "RH (%)", "Ramp (s)", "RPM", "Accel (RPM/s)", "Time (s)", "Mobility", "On/Off", "Vt", "S.T.S") -> (→"Transformer \nHeaders":string[])
